vi "main.vi"() -> ()   [LabVIEW 2020]
uses:
  DataCluster.ctl
  <vilib>/userDefined/High Color/IMAQdx.ctl
  <vilib>/vision/Image Controls.llb/IMAQ Image.ctl
  <vilib>/Platform/TimedLoop/XDataNode/timing_clust.ctl
  <vilib>/Platform/TimedLoop/XDataNode/nitl_modes.ctl
  <vilib>/Platform/TimedLoop/XDataNode/wakeup.ctl
  <vilib>/DAQmx/write.llb/DAQmx Write (Analog DBL 1Chan 1Samp).vi
  <extravilib>/ChannelInstances/Tag-t'DataCluster.ctl'/Read With Abort.vi
  <extravilib>/ChannelInstances/Tag-c(a[.](dbl),a[.](dbl))/Write With Abort.vi
  <extravilib>/ChannelInstances/Tag-str/Write With Abort.vi
  <extravilib>/ChannelInstances/Tag-str/Read With Abort.vi
  <extravilib>/ChannelInstances/Tag-t'DataCluster.ctl'/Write With Abort.vi
  <extravilib>/ChannelInstances/Tag-c(a[.](dbl),a[.](dbl))/Instantiate.vi
  <extravilib>/ChannelInstances/Tag-str/Instantiate.vi
  <extravilib>/ChannelInstances/Tag-t'DataCluster.ctl'/Instantiate.vi
  <extravilib>/ChannelInstances/Tag-t'DataCluster.ctl'/EndpointRead.vi
  <extravilib>/ChannelInstances/Tag-c(a[.](dbl),a[.](dbl))/Endpoint.vi
  <extravilib>/ChannelInstances/Tag-str/Endpoint.vi
  <vilib>/DAQmx/create/channels.llb/DAQmx Create Channel (AI-Voltage-Basic).vi
  <vilib>/DAQmx/create/channels.llb/DAQmx Create Channel (AO-Voltage-Basic).vi
  <vilib>/DAQmx/miscellaneous.llb/DAQmx Fill In Error Info.vi
  <extravilib>/ChannelInstances/Tag-str/EndpointRead.vi
  <extravilib>/ChannelInstances/Tag-t'DataCluster.ctl'/Endpoint.vi
  <vilib>/platform/TimedLoop/XDataNode/XDataNode.xnode
  <vilib>/vision/driver/NI_Vision_Acquisition_Software.lvlib
  <extravilib>/ChannelInstances/Tag-t'DataCluster.ctl'.lvlib
  <vilib>/Platform/TimedLoop/XDataNode/XDNodeRunTimeDep.lvlib
  <resource>/objmgr/daqmx.rc
  <extravilib>/ChannelInstances/Tag-str.lvlib
  <extravilib>/ChannelInstances/Tag-c(a[.](dbl),a[.](dbl)).lvlib
panel:
  out "version":string="version 0.0.0.1" caption="Version"
  in  "Start":bool
  out "Title":string="Ice Nucleation Setup" caption="Version"
  in  "Help":bool
  out "Temps":waveform(dbl)[](graph)
  out "Gradients":waveform(dbl)[](graph)
  out "Camera Feed":T1(plugin-control)
  out "Period (ms)":i64
  out "Output%":dbl(slide) caption="Peltier Output" scale=0.0..100.0
  out "StatusString":string="Closing System"
  # "Camera Feed"
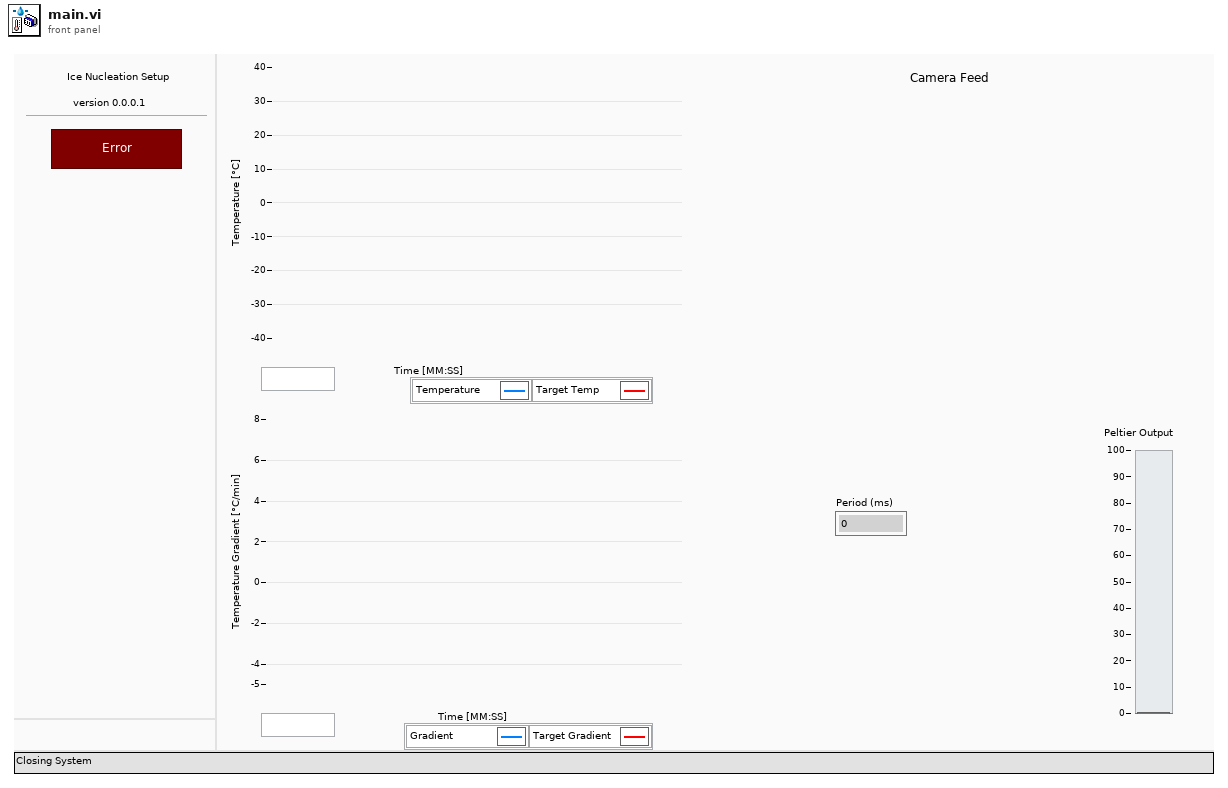
[diagram p1: front panel]
types:
  T1 = typedef "IMAQ Image.ctl" = refnum<image>
  T2 = typedef "DataCluster.ctl" = cluster{"Core":cluster{"Current VI Reference":refnum<vi>, "Close Panel on Exit?":bool, "Exit":bool}, "Connections":cluster{"cDAQ Therm":cluster{"Task":refnum<k21>, "Connected":bool, "Active":bool}, "cDAQ Voltage":cluster{"Task":refnum<k21>, "Connected":bool, "Active":bool}, "Camera":cluster{"Session":T3, "Connected":bool, "Active":bool}}, "Data Acquisition":cluster{"Setup":cluster{"Label":string, "Operator":string, "Notes":string, "TempGrad":dbl, "TargetTemp":dbl, "Sample Volume":dbl}, "Camera":cluster{"Image":T1, "Save Image":T1, "Image Frequency":i32, "Rectangle":T4}, "Thermistor":cluster{"Sample Size":i32, "Calibration":cluster{"B0.100":dbl[], "R25":dbl[], "c":dbl[][], "State":bool[], "V_S":dbl, "R_S":dbl}, "Timing Mode":i32}, "Partition":cluster{"Data":string[][], "Cell Label":string, "Cell Color":u32, "Height":i32, "Width":i32, "Grid":string[][]}, "Queue":cluster{"Size":i32, "Queue":refnum<queue>}, "Sample Rate":i32, "Active":bool, "Ready":bool, "Graph Mode":u16}, "Control":cluster{"Sample Rate":i32, "PID gains":cluster{"proportional gain (Kc)":dbl, "integral time (Ti, min)":dbl, "derivative time (Td, min)":dbl}}}
  T3 = typedef "IMAQdx.ctl" = refnum<k21>
  T4 = typedef "IMAQ Rectangle" = cluster{"Left":i32, "Top":i32, "Right":i32, "Bottom":i32, "Rotation":dbl}
  T5 = enum32{"Invalid", "Standard", "Closed", "Hidden", "Minimized", "Maximized"}
  T6 = enum32{"invalid app kind", "Development System", "Run Time System", "Student Edition", "Embedded LabVIEW", "Evaluation", "Custom"}
  T7 = cluster{"cDAQ Therm":cluster{"Task":refnum<k21>, "Connected":bool, "Active":bool}, "cDAQ Voltage":cluster{"Task":refnum<k21>, "Connected":bool, "Active":bool}, "Camera":cluster{"Session":T3, "Connected":bool, "Active":bool}}
  T8 = enum8{"Enabled", "Disabled", "Disabled and Grayed Out"}
  T9 = cluster{"Current VI Reference":refnum<vi>, "Close Panel on Exit?":bool, "Exit":bool}
  T10 = typedef "Tag-t'DataCluster.ctl'.lvlib/))Channel.ctl" = refnum<queue>
  T11 = typedef "XDNodeRunTimeDep.lvlib/timing_clust.ctl" = cluster{"Expected End [f-1]":u64, "Actual End [f-1]":u64, "Finished Late? [f-1]":bool, "Expected End [i-1]":u64, "Actual End [i-1]":u64, "Finished Late? [i-1]":bool, "Expected Start [i]":u64, "Actual Start [i]":u64, "Expected Start [f]":u64, "Actual Start [f]":u64, "Source Name":string, "Structure Name":string, "Period":i64, "Deadline":i64, "Offset":i64, "Start":i64, "Priority":i32, "Timeout":i32, "Mode":T12, "Wakeup Reason":T13, "Error":errorcluster, "Source Type":string, "Secondary Source Type":string, "Global End Time":u64, "Global Start Time":u64, "Frame Duration":u64, "Iteration Duration":u64, "Assigned CPU":i32, "I/O Scan Engine Mode":u32}
  T12 = typedef "XDNodeRunTimeDep.lvlib/nitl_modes.ctl" = enum32{"No Change", "Process missed periods, maintain original phase", "Discard missed periods, maintain original phase", "Process missed periods, ignore original phase", "Discard missed periods, ignore original phase"}
  T13 = typedef "XDNodeRunTimeDep.lvlib/wakeup.ctl" = enum32{"Normal", "Aborted", "Asynchronous wakeup", "Timing source error", "Timed loop error", "Timeout"}
  T14 = typedef "Tag-str.lvlib/))Channel.ctl" = refnum<queue>
  T15 = cluster{"Temperature Readings Duplicate":dbl[], "Voltage Readings Duplicate":dbl[]}
  T16 = typedef "Tag-c(a[.](dbl),a[.](dbl)).lvlib/))Channel.ctl" = refnum<queue>
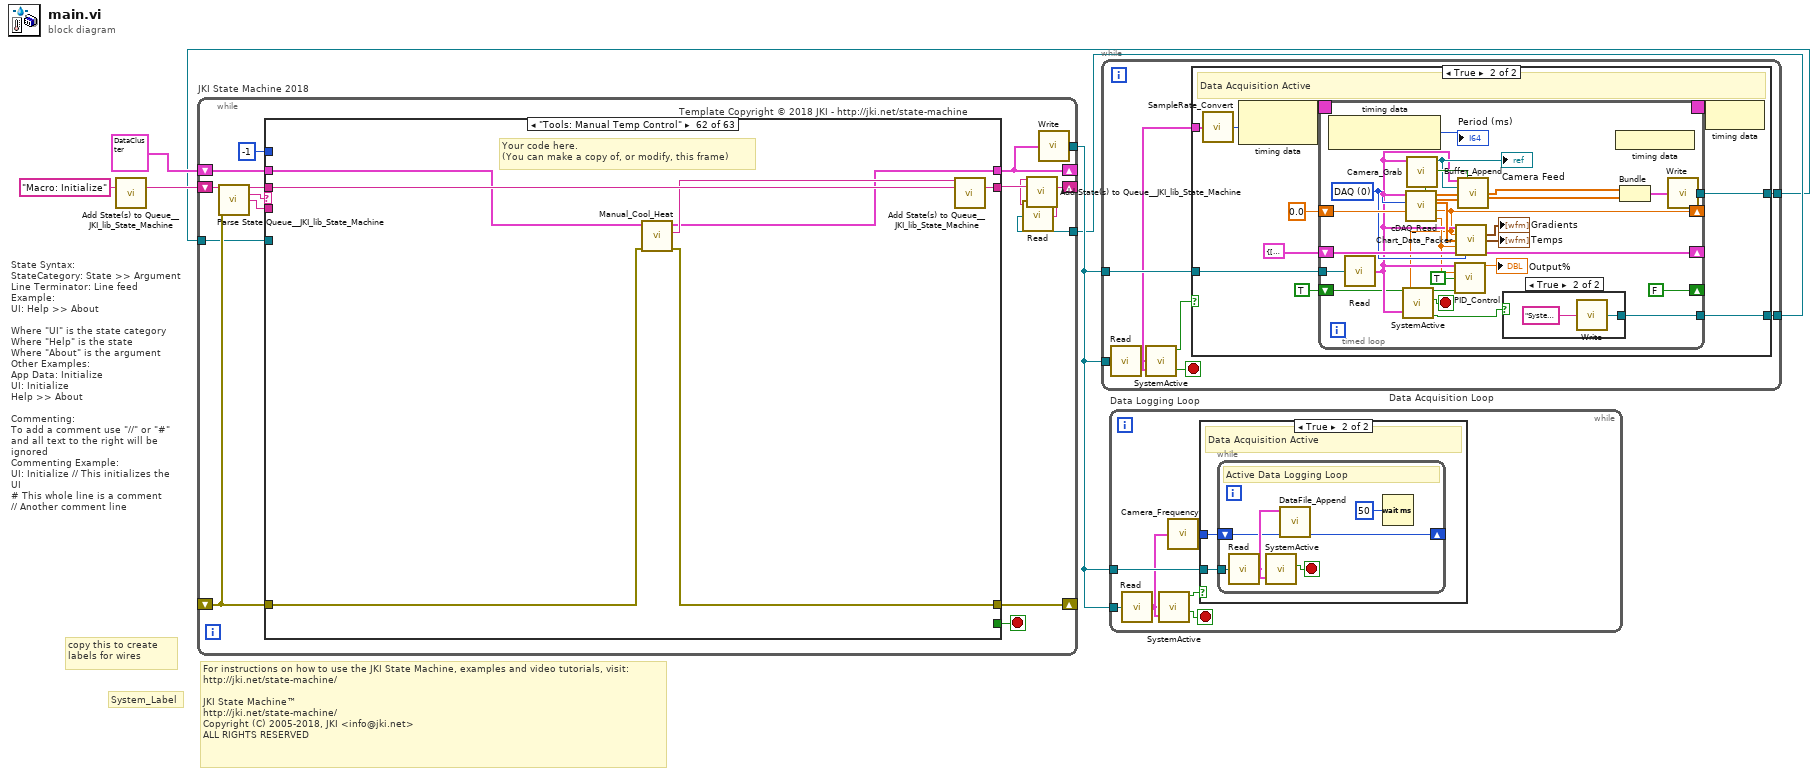
[diagram p0: block diagram]
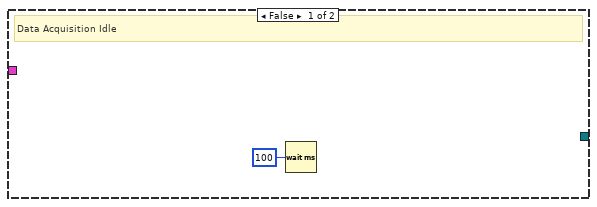
[diagram p2: hidden frame]
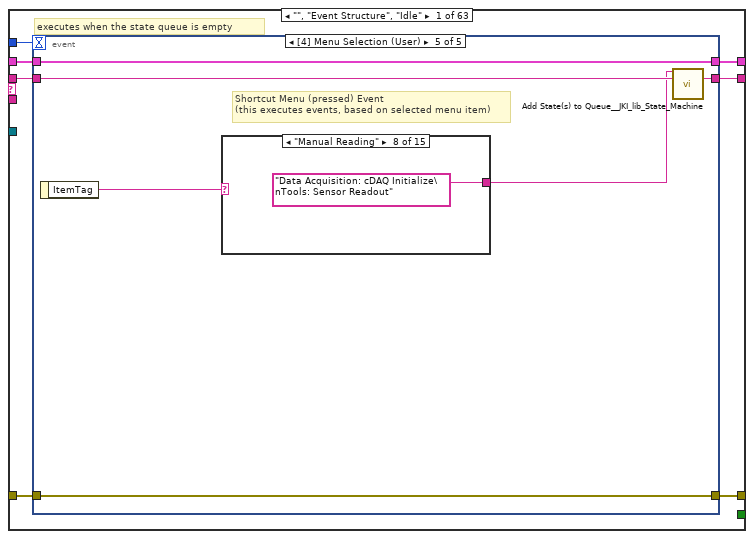
[diagram p4: hidden frame]
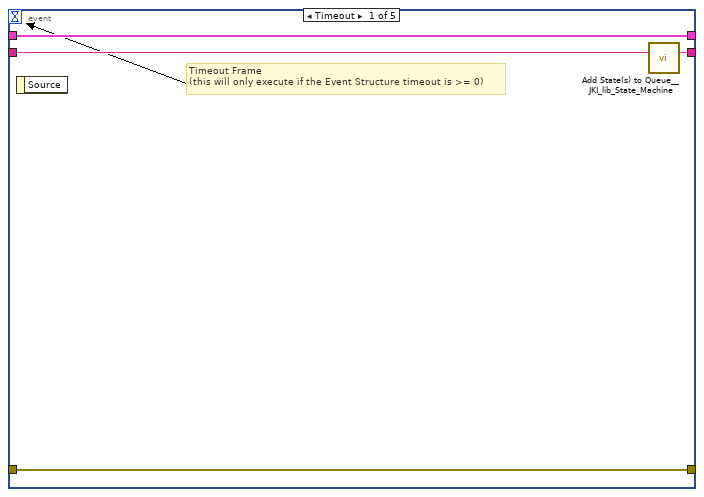
[diagram p5: hidden frame]
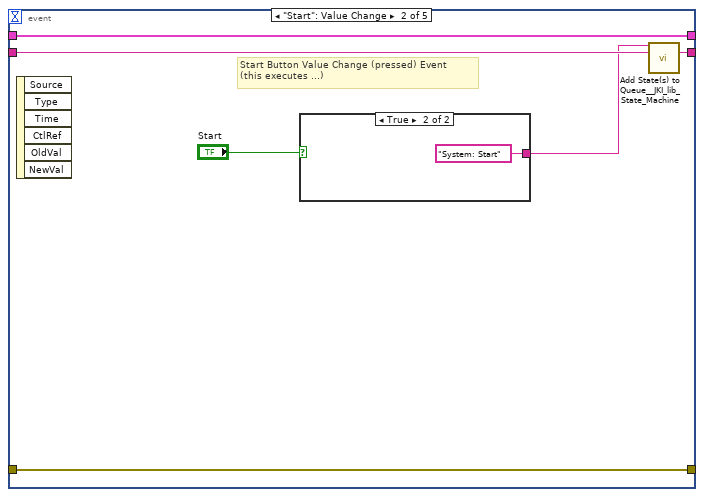
[diagram p6: hidden frame]
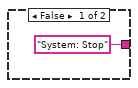
[diagram p7: hidden frame]
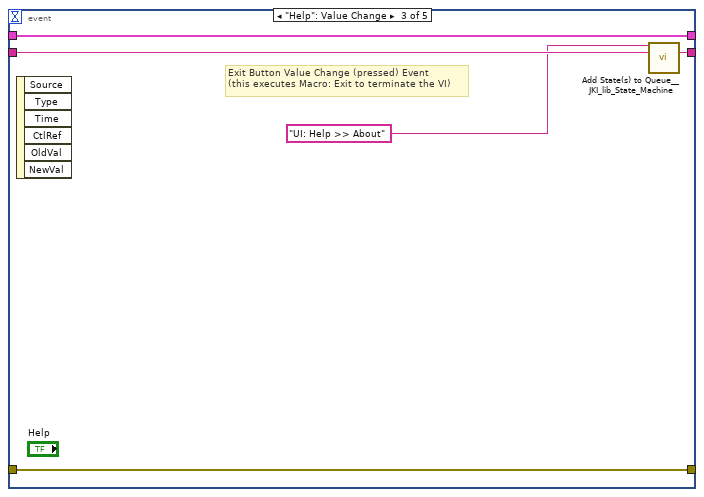
[diagram p8: hidden frame]
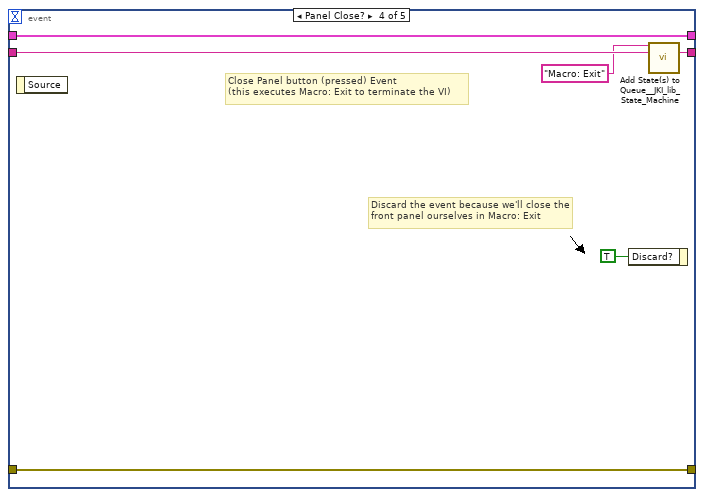
[diagram p9: hidden frame]
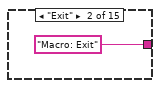
[diagram p11: hidden frame]
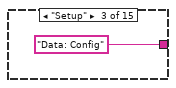
[diagram p12: hidden frame]
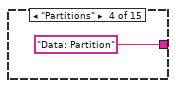
[diagram p13: hidden frame]
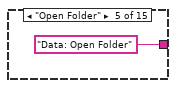
[diagram p14: hidden frame]
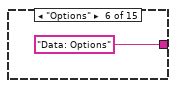
[diagram p15: hidden frame]
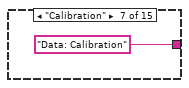
[diagram p16: hidden frame]
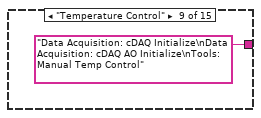
[diagram p17: hidden frame]
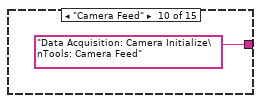
[diagram p18: hidden frame]
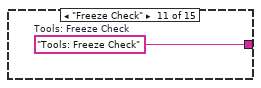
[diagram p19: hidden frame]
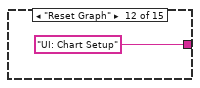
[diagram p20: hidden frame]
diagram:
  # "For instructions on how to use the JKI State Machine, examples and video tutorials, visit:\nhttp://jki.net/state-machine/\n\nJKI State Machine™\nhttp://jki.net/state-machine/\nCopyright (C) 2005-2018, JKI <info@jki.net>\nALL RIGHTS RESERVED"
  # "State Syntax:\nStateCategory: State >> Argument\nLine Terminator: Line feed\nExample:\nUI: Help >> About\n\nWhere \"UI\" is the state category\nWhere \"Help\" is the state\nWhere \"About\" is the argument\nOther Examples:\nApp Data: Initialize\nUI: Initialize\nHelp >> About\n\nCommenting:\nTo add a comment use \"//\" or \"#\" and all text to the right will be ignored\nCommenting Example:\nUI: Initialize // This initializes the UI\n# This whole line is a comment\n// Another comment line"
  # "copy this to create labels for wires"
  # "System_Label"
  n1 = call <vilib>:"Add State(s) to Queue__JKI_lib_State_Machine.vi"("State(s) in (\"\")"="Macro: Initialize") -> ("States Out"=w6:string)  [unwired: 14 in]
  n2 = while "JKI State Machine 2018" {
    shift-right: [w13] -> _
    shift-left: T2 {"Core"={"Current VI Reference"=refnum, "Close Panel on Exit?"=FALSE, "Exit"=FALSE}, "Connections"={"cDAQ Therm"={"Task"="", "Connected"=FALSE, "Active"=FALSE}, "cDAQ Voltage"={"Task"="", "Connected"=FALSE, "Active"=FALSE}, "Camera"={"Session"="", "Connected"=FALSE, "Active"=FALSE}}, "Data Acquisition"={"Setup"={"Label"="", "Operator"="", "Notes"="", "TempGrad"=0.0, "TargetTemp"=0.0, "Sample Volume"=1.0}, "Camera"={"Image"=refnum, "Save Image"=refnum, "Image Frequency"=20, "Rectangle"={"Left"=0, "Top"=0, "Right"=0, "Bottom"=0, "Rotation"=0.0}}, "Thermistor"={"Sample Size"=0, "Calibration"={"B0.100"=[], "R25"=[], "c"=[], "State"=[], "V_S"=0.0, "R_S"=0.0}, "Timing Mode"=14713}, "Partition"={"Data"=[], "Cell Label"="", "Cell Color"=0, "Height"=10, "Width"=16, "Grid"=[]}, "Queue"={"Size"=0, "Queue"=refnum}, "Sample Rate"=0, "Active"=FALSE, "Ready"=FALSE, "Graph Mode"=0}, "Control"={"Sample Rate"=0, "PID gains"={"proportional gain (Kc)"=0.0, "integral time (Ti, min)"=0.0, "derivative time (Td, min)"=0.0}}} ("DataCluster") -> [w16]
    shift-right: [w18] -> _
    shift-left: _ -> [w14]
    shift-right: [w10] -> _
    shift-left: w6 -> [w19]
    tunnel: [w12] -> w3
    tunnel: w2 -> [w9]
    tunnel: w1 -> [w7]
    stop <- w17 stop-if-true
    # "Template Copyright © 2018 JKI - http://jki.net/state-machine"
    n3 = call <vilib>:"Parse State Queue__JKI_lib_State_Machine.vi"("State Queue"=w19, "Error In (no error)"=w14) -> ("Remaining States"=w21:string, "Current State"=w22:string, "Arguments"=w20:string)  [unwired: 11 in]
    n4 = case shown="\"Tools: Manual Temp Control\"" w22 {
      selector: w22 -> [_ _ w77 _ _ _ _ _ _ _ _ _ _ _ _ _ _ _ _ _ _ _ _ _ _ _ _ _ _ _ _ _ _ _ _ _ _ _ _ _ _ _ _ _ _ _ _ _ _ _ _ _ _ _ _ _ _ _ _ _ _ _ _]
      tunnel: w21 -> [w29 w76 w81 w100 w106 w113 w117 w127 w134 w139 w144 w150 w156 w163 w168 w174 w180 w185 w209 w223 w238 w246 w251 w264 w282 w300 w314 w322 w338 w354 w372 w384 w394 w408 w413 w418 w423 w434 w442 w457 w468 w537 w542 w553 w557 w566 w579 w586 w596 w607 w623 w639 w655 w673 w689 w707 w714 w724 w737 w744 w750 w757 w761]
      tunnel: w20 -> [_ _ _ _ _ _ _ _ _ _ _ _ _ _ _ _ _ _ _ _ _ _ _ _ _ _ _ _ _ _ _ _ _ _ _ w414 w419 _ w438 w452 w462 _ _ _ _ _ _ _ _ _ _ _ _ _ _ _ _ _ _ _ _ _ _]
      tunnel: w16 -> [w27 w73 w79 w93 w103 w109 w114 _ w131 w136 w141 w148 w153 w161 w164 w172 w176 w183 w195 w217 w227 w243 w248 w254 w280 w298 w311 w318 w334 w350 w365 w381 w392 w406 w411 w416 w421 w431 w440 w455 w464 w534 w539 w550 w554 w558 w576 w581 w593 w602 w618 w634 w650 w668 w685 w705 w708 w715 w734 w742 w748 w755 w758]
      tunnel: [w26 w74 w83 w97 errorcluster {"status"=FALSE, "code"=0, "source"=""} ("error out") w111 w115 w118 w128 w137 w142 w145 w154 w158 w165 w170 w178 w181 w193 w210 w225 w244 w249 w261 w277 w296 w312 w315 w331 w347 w370 w382 w391 w405 w410 w415 w420 w432 w439 w453 w465 w535 w540 w551 w555 w564 w577 w584 w594 w603 w619 w635 w651 w669 w681 w703 w710 w717 w735 w740 w746 w753 w759] -> w18
      tunnel: w14 -> [w25 w74 w82 w97 w102 w111 w115 w119 w130 w137 w142 w145 w154 w159 w166 w171 w177 w182 w187 w211 w226 w244 w249 w260 w275 w295 w312 w316 w332 w348 w370 w382 w391 w405 w410 w415 w420 w432 w439 w454 w466 w535 w540 w551 w555 w564 w577 w584 w594 w604 w620 w636 w652 w670 w686 w704 w711 w717 w735 w741 w747 w754 w759]
      tunnel: [w28 w75 w80 w99 w105 w112 w116 w126 w133 w138 w143 w149 w155 w162 w167 w173 w179 w184 w208 w222 w237 w245 w250 w263 w281 w299 w313 w321 w337 w353 w371 w383 w393 w407 w412 w417 w422 w433 w441 w456 w467 w536 w541 w552 w556 w565 w578 w585 w595 w606 w622 w638 w654 w672 w688 w706 w713 w723 w736 w743 w749 w756 w760] -> w11
      tunnel: [_ _ _ _ _ TRUE _ _ _ _ _ _ _ _ _ _ _ _ _ _ _ _ _ _ _ _ _ _ _ _ _ _ _ _ _ _ _ _ _ _ _ _ _ _ _ _ _ _ _ _ _ _ _ _ _ _ _ _ _ _ _ _ _] -> w17
      tunnel: [w24 w73 w79 w98 w103 w107 w114 w125 w131 w135 w140 w147 w152 w160 w164 w169 w175 w183 w195 w217 w227 w243 w248 w262 w279 w297 w311 w317 w333 w349 w364 w381 w392 w406 w411 w416 w421 w431 w440 w455 w464 w534 w539 w550 w554 w558 w575 w580 w593 w601 w617 w633 w649 w671 w684 w702 w708 w719 w734 w742 w748 w751 w758] -> w13
      tunnel: -1 ("Timeout") -> [w23 _ _ _ _ _ _ _ _ _ _ _ _ _ _ _ _ _ _ _ _ _ _ _ _ _ _ _ _ _ _ _ _ _ _ _ _ _ _ _ _ _ _ _ _ _ _ _ _ _ _ _ _ _ _ _ _ _ _ _ _ _ _]
      tunnel: w7 -> [_ _ _ _ _ _ _ _ _ _ _ _ _ _ _ _ _ _ _ _ _ _ _ _ _ _ _ _ _ _ _ _ _ _ _ _ _ _ _ _ _ _ _ _ _ _ _ _ _ _ _ _ _ _ _ _ _ _ _ w739 _ _ _]
      frame "", "Event Structure", "Idle" {
        # "executes when the state queue is empty"
        n5 = event shown="[4] Menu Selection (User)" {
          selector: _ -> [_ _ _ _ _]
          dyn-events: _ -> [_ _ _ _ _]
          timeout: w23 -> [_ _ _ _ _]
          tunnel: w29 -> [w33 w39 w46 w52 w58]
          tunnel: [w32 w38 w45 w51 w57] -> w28
          tunnel: w27 -> [w30 w36 w43 w49 w55]
          tunnel: [w31 w37 w44 w50 w56] -> w26
          tunnel: w25 -> [w31 w37 w44 w50 w56]
          tunnel: [w30 w36 w43 w49 w55] -> w24
          event Timeout {
            # "Timeout Frame\n(this will only execute if the Event Structure timeout is >= 0)"
            n6 = event-data() -> ()  [unwired: 1 in, 1 out]
            n7 = call <vilib>:"Add State(s) to Queue__JKI_lib_State_Machine.vi"("State(s) in (\"\")"=w33) -> ("States Out"=w32:string)  [unwired: 14 in]
          }
          event "Start": Value Change {
            # "Start Button Value Change (pressed) Event\n(this executes ...)"
            n8 = event-data() -> ()  [unwired: 1 in, 6 out]
            n9 = case shown="True" "Start" {
              tunnel: ["System: Stop" ("State(s) in Front (\"\")") "System: Start" ("State(s) in Front (\"\")")] -> w34
              frame False {
              }
              frame True {
              }
            }
            n10 = call <vilib>:"Add State(s) to Queue__JKI_lib_State_Machine.vi"("State(s) in Front (\"\")"=w34, "State(s) in (\"\")"=w39) -> ("States Out"=w38:string)  [unwired: 13 in]
          }
          event "Help": Value Change {
            # "Exit Button Value Change (pressed) Event\n(this executes Macro: Exit to terminate the VI)"
            n11 = event-data() -> ()  [unwired: 1 in, 6 out]
            n12 = call <vilib>:"Add State(s) to Queue__JKI_lib_State_Machine.vi"("State(s) in Front (\"\")"="UI: Help >> About" ("State(s) in Front (\"\")"), "State(s) in (\"\")"=w46) -> ("States Out"=w45:string)  [unwired: 13 in]
          }
          event Panel Close? {
            # "Discard the event because we'll close the front panel ourselves in Macro: Exit"
            # "Close Panel button (pressed) Event\n(this executes Macro: Exit to terminate the VI)"
            n13 = event-data() -> ()  [unwired: 1 in, 1 out]
            n14 = event-data("Discard?"=TRUE) -> ()  [unwired: 1 in, 1 out]
            n15 = call <vilib>:"Add State(s) to Queue__JKI_lib_State_Machine.vi"("State(s) in Front (\"\")"="Macro: Exit", "State(s) in (\"\")"=w52) -> ("States Out"=w51:string)  [unwired: 13 in]
          }
          event Menu Selection (User) {
            # "Shortcut Menu (pressed) Event\n(this executes events, based on selected menu item)"
            n16 = event-data() -> ("ItemTag"=w54:string)  [unwired: 1 in]
            n17 = case shown="\"Manual Reading\"" w54 {
              tunnel: [_ "Macro: Exit" "Data: Config" "Data: Partition" "Data: Open Folder" "Data: Options" "Data: Calibration" "Data Acquisition: cDAQ Initialize\nTools: Sensor Readout" "Data Acquisition: cDAQ Initialize\nData Acquisition: cDAQ AO Initialize\nTools: Manual Temp Control" "Data Acquisition: Camera Initialize\nTools: Camera Feed" w68 "UI: Chart Setup" "UI: Cursor Set >> Busy\nConnections: Terminate\nConnections: Initialize\nUI: Cursor Set >> Idle" "System: Override" "UI: Connections Status"] -> w53
              frame "False", Default {
              }
              frame "Exit" {
              }
              frame "Setup" {
              }
              frame "Partitions" {
              }
              frame "Open Folder" {
              }
              frame "Options" {
              }
              frame "Calibration" {
              }
              frame "Manual Reading" {
              }
              frame "Temperature Control" {
              }
              frame "Camera Feed" {
              }
              frame "Freeze Check" {
                w68 = "Tools: Freeze Check"  # Tools: Freeze Check
              }
              frame "Reset Graph" {
              }
              frame "Reconnect" {
              }
              frame "System Override" {
              }
              frame "Status" {
              }
            }
            n18 = call <vilib>:"Add State(s) to Queue__JKI_lib_State_Machine.vi"("State(s) in Front (\"\")"=w53, "State(s) in (\"\")"=w58) -> ("States Out"=w57:string)  [unwired: 13 in]
          }
        }
      }
      frame "---------- Core ----------" {
        # "Do not put any code in this frame.\n(it is a separator no-op)"
        n19 = call <vilib>:"Add State(s) to Queue__JKI_lib_State_Machine.vi"("State(s) in (\"\")"=w76) -> ("States Out"=w75:string)  [unwired: 14 in]
      }
      frame Default {
        w86 = 42 items=["No error", "Argument error", "Memory is full", "Out of zone", "End of file", "File already open", "Generic file I/O error", "File not found", "File permission error", "Disk is full", "Duplicate path", "Too many files open", "System feature not enabled", "Resource file not found", "Cannot add resource", "Resource not found", "Image not found", "Image memory error", "Pen does not exist", "Config type invalid", "Config token not found", "Config parse error", "Config memory error", "Bad external code format", "Bad external code offset", "External code not present", "Null window", "Destroy window error", "Null menu", "Print aborted", "Bad print record", "Print driver error", "Windows error during printing", "Memory error during printing", "Print dialog error", "Generic print error", "Invalid device refnum", "Device not found", "Device parameter error", "Device unit error", "Cannot open device", "Device call aborted", "Generic error", "Cancelled by user", "Object ID too low", "Object ID too high", "Object not in heap", "Unknown heap", "Unknown object (invalid DefProc)", "Unknown object (DefProc not in table)", "Message out of range", "Invalid (null) method", "Unknown message", "Manager call not supported", "Bad address", "Network operation in progress", "Network operation timed out", "Connection is busy", "Network attribute not supported", "Network error", "Address in use", "System out of memory", "Connection aborted", "Connection refused", "Not connected", "Already connected", "Connection closed", "Initialization error (interapplication manager)", "Bad occurrence", "Wait on unbound occurrence handler", "Occurrence queue overflow", "Datalog type conflict", "Unused", "Unrecognized type (interapplication manager)", "Memory corrupt", "Failed to make temporary DLL", "Old CIN version", "Drag socket not found", "Failed to load drop-object", "Failed to register OLE object", "Failed to release OLE object", "Format specifier type mismatch", "Unknown format specifier", "Too few format specifiers", "Too many format specifiers", "Scan failed", "Newer CIN version", "Error converting to variant", "Runtime menu error", "Password tampered", "Variant attribute not found", "Incompatible variant data type", "Event data is not available", "Event Store is not present", "Occurrence is not found", "Event Queue is not created", "Event info is not available", "Refnum passed is NULL", "Error retrieving Class GUID", "Error retrieving CoClass GUID", "Error retrieving TypeLib GUID.", "Bad built application magic bytes.", "Specific driver is different from the specific driver associated with the Logical Name.", "There is no session opened to the class driver.", "Max Error", "MAX - Error with config objects", "MAX - Error loading configuration", "MAX - Group not supported"]
        # "Current State"
        # "Do not delete, rename, or modify this frame.\n(this is used to capture unhandled states and typos)"
        # "Handle mistyped state name (developer tool)"
        n20 = Format Into String(format string="Software Exception: Unhandled State \"%s\"." ("message"), error in=w82, w77) -> (resulting string=w85:string, error out=w84:errorcluster)  [unwired: 1 in]
        n21 = call <vilib>:"Error Cluster From Error Code.vi"("show call chain? (False)"=TRUE, "error in (no error)"=w84, "error message (\"\")"=w85, "error code (0)"=w86) -> ("error out"=w83:errorcluster)  [unwired: 5 in]
        n22 = call <vilib>:"Add State(s) to Queue__JKI_lib_State_Machine.vi"("State(s) in (\"\")"=w81) -> ("States Out"=w80:string)  [unwired: 14 in]
      }
      frame "Initialize Core Data" {
        # "Do not delete, rename, or modify this frame.\n(this is used to determine panel behavior on exit)"
        # "originally closed?"
        # "exe?"
        # "If panel starts closed or is an EXE, then close it when we exit"
        n23 = property class="VI"() -> ("FP.State"=w90:T5)  [unwired: 2 in, 2 out]
        n24 = property class="App"() -> ("App.Kind"=w96:T6)  [unwired: 2 in, 2 out]
        n25 = control-ref of="Current VI Reference"() -> (w91:refnum<vi>)
        n26 = Equal?(x=w90, y=T5."Closed" ("Front Panel Window:State")) -> (x = y?=w88:bool)
        n27 = Equal?(x=w96, y=T6."Run Time System" ("Application:Kind")) -> (x = y?=w94:bool)
        n28 = Or(x=w88, y=w94) -> (x .or. y?=w92:bool)
        n29 = Bundle By Name(cluster=w93, "Core.Current VI Reference"=w91, "Core.Close Panel on Exit?"=w92) -> (w98:T2)
        n30 = call <vilib>:"Add State(s) to Queue__JKI_lib_State_Machine.vi"("State(s) in (\"\")"=w100) -> ("States Out"=w99:string)  [unwired: 14 in]
      }
      frame "Error Handler" {
        # "Unhandled Error -- Display it"
        # "Handle any errors here.\nYou can also output any states to clean-up after errors occur"
        # "Clear error"
        n31 = call <vilib>:"General Error Handler.vi"("error in (no error)"=w102) -> ()  [unwired: 10 in, 5 out]
        n32 = call <vilib>:"Add State(s) to Queue__JKI_lib_State_Machine.vi"("State(s) in Front (\"\")"="/* Post Error States", "State(s) in (\"\")"=w106) -> ("States Out"=w105:string)  [unwired: 13 in]
      }
      frame "Exit" {
        # "Do not put any code in this frame.\n(No errors that occur here will be handled.)"
        n33 = Bundle By Name(cluster=w109, "Core.Exit"=TRUE) -> (w107:T2)
        n34 = call <vilib>:"Add State(s) to Queue__JKI_lib_State_Machine.vi"("State(s) in (\"\")"=w113) -> ("States Out"=w112:string)  [unwired: 14 in]
      }
      frame "---------- Data ----------" {
        # "Do not put any code in this frame.\n(It is a separator no-op. You can make a copy of this frame to create a new Data frame)"
        n35 = call <vilib>:"Add State(s) to Queue__JKI_lib_State_Machine.vi"("State(s) in (\"\")"=w117) -> ("States Out"=w116:string)  [unwired: 14 in]
      }
      frame "Data: Initialize" {
        w124 = T9 {"Current VI Reference"=refnum, "Close Panel on Exit?"=FALSE, "Exit"=FALSE}  # Core
        # "Initialize the shift-register data, here.\n(data names are defined by what you wire into the bundle function)"
        n36 = call "Settings_Load.vi"("error in"=w119) -> ("error out"=w120:errorcluster, "DataCluster out"=w121:T2)  [unwired: 9 in]
        n37 = call "Settings_Save.vi"("error in"=w120, "DataCluster"=w121) -> ("error out"=w118:errorcluster)  [unwired: 9 in]
        n38 = Bundle By Name(cluster=w121, "Core"=w124, "Connections"=T7 {"cDAQ Therm"={"Task"="ThermTask", "Connected"=FALSE, "Active"=FALSE}, "cDAQ Voltage"={"Task"="", "Connected"=FALSE, "Active"=FALSE}, "Camera"={"Session"="", "Connected"=FALSE, "Active"=FALSE}}, "Data Acquisition.Active"=FALSE ("System.Active")) -> (w125:T2)
        n39 = call <vilib>:"Add State(s) to Queue__JKI_lib_State_Machine.vi"("State(s) in (\"\")"=w127) -> ("States Out"=w126:string)  [unwired: 14 in]
      }
      frame "Data: Cleanup" {
        # "Cleanup any data and references, here.\n(this is called automatically, by the Macro: Exit)"
        n40 = Unbundle By Name(w131) -> ("Core.Current VI Reference"=w132:refnum<vi>)
        n41 = call "Settings_Save.vi"("error in"=w130, "DataCluster"=w131) -> ("error out"=w129:errorcluster)  [unwired: 9 in]
        n42 = Close Reference(reference=w132, error in (no error)=w129) -> (error out=w128:errorcluster)
        n43 = call <vilib>:"Add State(s) to Queue__JKI_lib_State_Machine.vi"("State(s) in (\"\")"=w134) -> ("States Out"=w133:string)  [unwired: 14 in]
      }
      frame "Data: Config" {
        # "Access Data Setup here.\n(this is called automatically, by the Settings Event Run time menu)"
        n44 = call "Settings_Config.vi"("DataCluster in"=w136) -> ("DataCluster out"=w135:T2)  [unwired: 10 in]
        n45 = call <vilib>:"Add State(s) to Queue__JKI_lib_State_Machine.vi"("State(s) in (\"\")"=w139) -> ("States Out"=w138:string)  [unwired: 14 in]
      }
      frame "Data: Partition" {
        # "Access Data Setup here.\n(this is called automatically, by the Settings Event Run time menu)"
        n46 = call "Partition_Setup.vi"("DataCluster in"=w141) -> ("DataCluster out"=w140:T2)  [unwired: 9 in, 1 out]
        n47 = call <vilib>:"Add State(s) to Queue__JKI_lib_State_Machine.vi"("State(s) in (\"\")"=w144) -> ("States Out"=w143:string)  [unwired: 14 in]
      }
      frame "Data: Options" {
        # "Access Data Setup here.\n(this is called automatically, by the Settings Event Run time menu)"
        n48 = call "Options.vi"("DataCluster in"=w148) -> ("State"=w146:string, "DataCluster out"=w147:T2)  [unwired: 9 in]
        n49 = call <vilib>:"Add State(s) to Queue__JKI_lib_State_Machine.vi"("State(s) in Front (\"\")"=w146, "State(s) in (\"\")"=w150) -> ("States Out"=w149:string)  [unwired: 13 in]
      }
      frame "Data: Calibration" {
        # "Access Data Setup here.\n(this is called automatically, by the Settings Event Run time menu)"
        n50 = call "Thermistor_Callibration.vi"("DataCluster in"=w153) -> ("State Out"=w151:string, "DataCluster out"=w152:T2)  [unwired: 9 in]
        n51 = call <vilib>:"Add State(s) to Queue__JKI_lib_State_Machine.vi"("State(s) in Front (\"\")"=w151, "State(s) in (\"\")"=w156) -> ("States Out"=w155:string)  [unwired: 13 in]
      }
      frame "Data: Load Calibration" {
        # "Access Data Setup here.\n(this is called automatically, by the Settings Event Run time menu)"
        n52 = call "Thermistor_Callibration_Load.vi"("error in"=w159, "DataCluster"=w161) -> ("error out"=w158:errorcluster, "State"=w157:string, "DataCluster out"=w160:T2)  [unwired: 7 in]
        n53 = call <vilib>:"Add State(s) to Queue__JKI_lib_State_Machine.vi"("State(s) in Front (\"\")"=w157, "State(s) in (\"\")"=w163) -> ("States Out"=w162:string)  [unwired: 13 in]
      }
      frame "Data: Save Calibration" {
        # "Access Data Setup here.\n(this is called automatically, by the Settings Event Run time menu)"
        n54 = call "Thermistor_Callibration_Save.vi"("error in"=w166, "DataCluster"=w164) -> ("error out"=w165:errorcluster)  [unwired: 9 in]
        n55 = call <vilib>:"Add State(s) to Queue__JKI_lib_State_Machine.vi"("State(s) in (\"\")"=w168) -> ("States Out"=w167:string)  [unwired: 14 in]
      }
      frame "Data: Setup File Config" {
        # "Access Data Setup here.\n(this is called automatically, by the Settings Event Run time menu)"
        n56 = call "SetupFile_Create.vi"("error in (no error)"=w171, "DataCluster"=w172) -> ("error out"=w170:errorcluster, "DataCluster out"=w169:T2)  [unwired: 8 in]
        n57 = call <vilib>:"Add State(s) to Queue__JKI_lib_State_Machine.vi"("State(s) in (\"\")"=w174) -> ("States Out"=w173:string)  [unwired: 14 in]
      }
      frame "Data: Stamp times" {
        # "Access Data Setup here.\n(this is called automatically, by the Settings Event Run time menu)"
        n58 = call "SetupFile_Stamp.vi"("error in (no error)"=w177, "DataCluster"=w176) -> ("error out"=w178:errorcluster, "DataCluster out"=w175:T2)  [unwired: 8 in]
        n59 = call <vilib>:"Add State(s) to Queue__JKI_lib_State_Machine.vi"("State(s) in (\"\")"=w180) -> ("States Out"=w179:string)  [unwired: 14 in]
      }
      frame "Data: Data File Config" {
        # "Access Data Setup here.\n(this is called automatically, by the Settings Event Run time menu)"
        n60 = call "DataFile_Create.vi"("error in (no error)"=w182, "DataCluster"=w183) -> ("error out"=w181:errorcluster)  [unwired: 9 in]
        n61 = call <vilib>:"Add State(s) to Queue__JKI_lib_State_Machine.vi"("State(s) in (\"\")"=w185) -> ("States Out"=w184:string)  [unwired: 14 in]
      }
      frame "Data: Files Unlock" {
        # "Access Data Setup here.\n(this is called automatically, by the Settings Event Run time menu)"
        n62 = Unbundle By Name(w195) -> ("Data Acquisition.Setup.Label"=w203:string)
        n63 = call <vilib>:"Application Directory.vi"() -> ("Application Directory"=w201:path)
        n64 = Path To String(path=w201) -> (string=w202:string)
        n65 = Concatenate Strings(w202, "\\Data\\", w203) -> (w188:string)
        n66 = Concatenate Strings(w188, "\\Partition.csv") -> (w191:string)
        n67 = Concatenate Strings(w188, "\\Setup.csv") -> (w205:string)
        n68 = Concatenate Strings(w188, "\\Data.csv") -> (w204:string)
        n69 = String To Path(string=w191) -> (path=w192:path)
        n70 = String To Path(string=w205) -> (path=w206:path)
        n71 = String To Path(string=w204) -> (path=w207:path)
        n72 = Set Permissions(7:i16 448 ("permissions"), 8:w187, 11:w192) -> (0:w186:errorcluster)  [unwired: 2 in, 1 out]
        n73 = Set Permissions(7:i16 448 ("permissions"), 8:w186, 11:w207) -> (0:w194:errorcluster)  [unwired: 2 in, 1 out]
        n74 = Set Permissions(7:i16 448 ("permissions"), 8:w194, 11:w206) -> (0:w193:errorcluster)  [unwired: 2 in, 1 out]
        n75 = call <vilib>:"Add State(s) to Queue__JKI_lib_State_Machine.vi"("State(s) in (\"\")"=w209) -> ("States Out"=w208:string)  [unwired: 14 in]
      }
      frame "Data: Open Folder" {
        # "Access Data Setup here.\n(this is called automatically, by the Settings Event Run time menu)"
        n76 = Unbundle By Name(w217) -> ("Data Acquisition.Setup.Label"=w221:string)
        n77 = call <vilib>:"Application Directory.vi"() -> ("Application Directory"=w219:path)
        n78 = Path To String(path=w219) -> (string=w220:string)
        n79 = Concatenate Strings(w220, "\\Data\\", w221) -> (w216:string)
        n80 = String To Path(string=w216) -> (path=w214:path)
        n81 = Format Into String(format string="cmd /c explorer.exe \"%s\"", w214) -> (resulting string=w213:string)  [unwired: 2 in, 1 out]
        n82 = call <vilib>:"System Exec.vi"("run minimized? (F)"=TRUE, "error in (no error)"=w211, "command line"=w213) -> ("error out"=w210:errorcluster)  [unwired: 5 in, 3 out]
        n83 = call <vilib>:"Add State(s) to Queue__JKI_lib_State_Machine.vi"("State(s) in (\"\")"=w223) -> ("States Out"=w222:string)  [unwired: 14 in]
      }
      frame "Data: Image Folder Setup" {
        # "Access Data Setup here.\n(this is called automatically, by the Settings Event Run time menu)"
        n84 = Unbundle By Name(w227) -> ("Data Acquisition.Setup.Label"=w229:string)
        n85 = call <vilib>:"Application Directory.vi"() -> ("Application Directory"=w236:path)
        n86 = Path To String(path=w236) -> (string=w235:string)
        n87 = Concatenate Strings(w235, "\\Data\\", w229, "\\Images\\" ("string")) -> (w233:string)
        n88 = String To Path(string=w233) -> (path=w232:path)
        n89 = call <vilib>:"Check if File or Folder Exists.vi"("error in (no error)"=w226, "path"=w232) -> ("error out"=w228:errorcluster, "file or folder exists?"=w231:bool, "dup path"=w230:path)  [unwired: 7 in]
        n90 = case shown="False" w231 {
          tunnel: w230 -> [w241 _]
          tunnel: w228 -> [w240 w242]
          tunnel: [w239 w242] -> w225
          frame False {
            n91 = Create Folder(path (use dialog)=w241, error in=w240) -> (error out=w239:errorcluster)  [unwired: 1 in, 2 out]
          }
          frame True {
          }
        }
        n92 = call <vilib>:"Add State(s) to Queue__JKI_lib_State_Machine.vi"("State(s) in (\"\")"=w238) -> ("States Out"=w237:string)  [unwired: 14 in]
      }
      frame "---------- Connections ----------" {
        # "Do not put any code in this frame.\n(It is a separator no-op. You can make a copy of this frame to create a new Data frame)"
        n93 = call <vilib>:"Add State(s) to Queue__JKI_lib_State_Machine.vi"("State(s) in (\"\")"=w246) -> ("States Out"=w245:string)  [unwired: 14 in]
      }
      frame "Connections: Initialize" {
        # "Initialize the System Connections, here.\n(this is called automatically, by the Macro: Init)"
        n94 = call <vilib>:"Add State(s) to Queue__JKI_lib_State_Machine.vi"("State(s) in Front (\"\")"="UI: StatusString >> Connecting cDAQ (Thermistors)\nConnections: Initialize cDAQ Therm\nUI: StatusString >> Connecting cDAQ Connection (Voltage Control)\nConnections: Initialize cDAQ AO\nUI: StatusString >> Connecting Camera\nConnections: Initialize Camera\nUI: StatusString >> Validating Connections\nConnections: Status" ("State(s) in Front (\"\")"), "State(s) in (\"\")"=w251) -> ("States Out"=w250:string)  [unwired: 13 in]
      }
      frame "Connections: Initialize cDAQ Therm" {
        w259 = 10106 items=["Default"=-1, "RSE"=10083, "NRSE"=10078, "Differential"=10106, "Pseudodifferential"=12529] ("input terminal configuration")
        # "Setup connection to cDAQs"
        # "Initialize the System Connections, here.\n(this is called automatically, by the Macro: Init)"
        n95 = Unbundle By Name(w254) -> ("Data Acquisition.Thermistor.Timing Mode"=w253:i32)
        n96 = call-poly <vilib>:"DAQmx Create Virtual Channel.vi"("input terminal configuration"=w259, "physical channels"="cDAQ1Mod2/ai3:0, cDAQ1Mod3/ai3:0", "error in"=w260) -> ("task out"=w258:refnum<k21>, "error out"=w257:errorcluster)  [unwired: 11 in]
        n97 = property class="DAQmx Channel"(reference=w258, error in=w257, "AI.ADCTimingMode"=w253) -> (reference out=w255:refnum<k21>, error out=w256:errorcluster)
        n98 = case shown="No Error" w256 {
          selector: w256 -> [w265 _]
          tunnel: w254 -> [w269 w273]
          tunnel: [w268 w272] -> w262
          tunnel: w255 -> [w266 _]
          tunnel: [w265 errorcluster {"status"=FALSE, "code"=0, "source"=""} ("error IO")] -> w261
          frame No Error {
            n99 = Bundle By Name(cluster=w269, "Connections.cDAQ Therm.Task"=w266, "Connections.cDAQ Therm.Connected"=TRUE ("Connections.cDAQ.Connected")) -> (w268:T2)
          }
          frame Error {
            n100 = Bundle By Name(cluster=w273, "Connections.cDAQ Therm.Connected"=FALSE ("Connections.cDAQ.Connected")) -> (w272:T2)
          }
        }
        n101 = call <vilib>:"Add State(s) to Queue__JKI_lib_State_Machine.vi"("State(s) in (\"\")"=w264) -> ("States Out"=w263:string)  [unwired: 14 in]
      }
      frame "Connections: Initialize cDAQ AO" {
        # "Setup connection to cDAQs"
        # "Initialize the System Connections, here.\n(this is called automatically, by the Macro: Init)"
        n102 = call-poly <vilib>:"DAQmx Create Virtual Channel.vi"("physical channels"="cDAQ1Mod1/ao0", "error in"=w275) -> ("task out"=w278:refnum<k21>, "error out"=w274:errorcluster)  [unwired: 12 in]
        n103 = case shown="Error .." w274 {
          selector: w274 -> [w283 _]
          tunnel: w280 -> [w287 w291]
          tunnel: [w286 w290] -> w279
          tunnel: w278 -> [w284 _]
          tunnel: [w283 errorcluster {"status"=FALSE, "code"=0, "source"=""} ("error IO")] -> w277
          frame No Error {
            n104 = Bundle By Name(cluster=w287, "Connections.cDAQ Voltage.Task"=w284, "Connections.cDAQ Voltage.Connected"=TRUE ("Connections.cDAQ.Connected")) -> (w286:T2)
          }
          frame Error {
            n105 = Bundle By Name(cluster=w291, "Connections.cDAQ Voltage.Connected"=FALSE ("Connections.cDAQ.Connected")) -> (w290:T2)
          }
        }
        n106 = call <vilib>:"Add State(s) to Queue__JKI_lib_State_Machine.vi"("State(s) in (\"\")"=w282) -> ("States Out"=w281:string)  [unwired: 14 in]
      }
      frame "Connections: Initialize Camera" {
        # "Setup connection to cDAQs"
        # "Initialize the System Connections, here.\n(this is called automatically, by the Macro: Init)"
        n107 = call <vilib>:"IMAQdx Open Camera.vi"("error in"=w295, "Session In"="16511205") -> ("error out"=w294:errorcluster, "Session Out"=w293:T3)  [unwired: 8 in]
        n108 = case shown="Error .." w294 {
          selector: w294 -> [w302 _]
          tunnel: w298 -> [w305 w309]
          tunnel: [w304 w308] -> w297
          tunnel: [w302 errorcluster {"status"=FALSE, "code"=0, "source"=""} ("error IO")] -> w296
          tunnel: w293 -> [w301 _]
          frame No Error {
            n109 = Bundle By Name(cluster=w305, "Connections.Camera.Session"=w301, "Connections.Camera.Connected"=TRUE ("Connections.cDAQ.Connected")) -> (w304:T2)
          }
          frame Error {
            n110 = Bundle By Name(cluster=w309, "Connections.Camera.Connected"=FALSE ("Connections.cDAQ.Connected")) -> (w308:T2)
          }
        }
        n111 = call <vilib>:"Add State(s) to Queue__JKI_lib_State_Machine.vi"("State(s) in (\"\")"=w300) -> ("States Out"=w299:string)  [unwired: 14 in]
      }
      frame "Connections: Terminate" {
        # "Terminate connection to DAQs and Power Supply (Peltier)"
        # "Terminate the System Connections, here.\n(this is called automatically, by the Macro: Exit)"
        n112 = call <vilib>:"Add State(s) to Queue__JKI_lib_State_Machine.vi"("State(s) in Front (\"\")"="UI: StatusString >> Terminating cDAQ Connection (Thermistors)\nConnections: Terminate cDAQ Therm\nUI: StatusString >> Terminating cDAQ Connection (Voltage Control)\nConnections: Terminate cDAQ AO\nUI: StatusString >> Terminating Camera Connection\nConnections: Terminate Camera" ("State(s) in Front (\"\")"), "State(s) in (\"\")"=w314) -> ("States Out"=w313:string)  [unwired: 13 in]
      }
      frame "Connections: Terminate cDAQ Therm" {
        # "Terminate connection to DAQs and Power Supply (Peltier)"
        # "Terminate the System Connections, here.\n(this is called automatically, by the Macro: Exit)"
        n113 = Unbundle By Name(w318) -> ("Connections.cDAQ Therm.Task"=w319:refnum<k21>, "Connections.cDAQ Therm.Connected"=w320:bool)
        n114 = case shown="True" w320 {
          tunnel: w319 -> [_ w330]
          tunnel: w318 -> [w324 w329]
          tunnel: [w324 w327] -> w317
          tunnel: w316 -> [w323 w326]
          tunnel: [w323 w325] -> w315
          frame False {
          }
          frame True {
            n115 = call <vilib>:"DAQmx Clear Task.vi"("task in"=w330, "error in"=w326) -> ("error out"=w325:errorcluster)  [unwired: 13 in]
            n116 = Bundle By Name(cluster=w329, "Connections.cDAQ Therm.Connected"=FALSE ("Connections.cDAQ.Connected")) -> (w327:T2)
          }
        }
        n117 = call <vilib>:"Add State(s) to Queue__JKI_lib_State_Machine.vi"("State(s) in (\"\")"=w322) -> ("States Out"=w321:string)  [unwired: 14 in]
      }
      frame "Connections: Terminate cDAQ AO" {
        # "Terminate connection to DAQs and Power Supply (Peltier)"
        # "Terminate the System Connections, here.\n(this is called automatically, by the Macro: Exit)"
        n118 = Unbundle By Name(w334) -> ("Connections.cDAQ Voltage.Task"=w335:refnum<k21>, "Connections.cDAQ Voltage.Connected"=w336:bool)
        n119 = case shown="True" w336 {
          tunnel: w335 -> [_ w346]
          tunnel: w334 -> [w340 w345]
          tunnel: [w340 w343] -> w333
          tunnel: w332 -> [w339 w342]
          tunnel: [w339 w341] -> w331
          frame False {
          }
          frame True {
            n120 = call <vilib>:"DAQmx Clear Task.vi"("task in"=w346, "error in"=w342) -> ("error out"=w341:errorcluster)  [unwired: 13 in]
            n121 = Bundle By Name(cluster=w345, "Connections.cDAQ Voltage.Connected"=FALSE ("Connections.cDAQ.Connected")) -> (w343:T2)
          }
        }
        n122 = call <vilib>:"Add State(s) to Queue__JKI_lib_State_Machine.vi"("State(s) in (\"\")"=w338) -> ("States Out"=w337:string)  [unwired: 14 in]
      }
      frame "Connections: Terminate Camera" {
        # "Terminate connection to DAQs and Power Supply (Peltier)"
        # "Terminate the System Connections, here.\n(this is called automatically, by the Macro: Exit)"
        n123 = Unbundle By Name(w350) -> ("Connections.Camera.Session"=w351:T3, "Connections.Camera.Connected"=w352:bool)
        n124 = case shown="False" w352 {
          tunnel: w351 -> [_ w359]
          tunnel: w350 -> [w356 w362]
          tunnel: [w356 w360] -> w349
          tunnel: w348 -> [w355 w358]
          tunnel: [w355 w357] -> w347
          frame False {
          }
          frame True {
            n125 = call <vilib>:"IMAQdx Close Camera.vi"("error in"=w358, "Session In"=w359) -> ("error out"=w357:errorcluster)  [unwired: 9 in]
            n126 = Bundle By Name(cluster=w362, "Connections.cDAQ Therm.Connected"=FALSE ("Connections.cDAQ.Connected")) -> (w360:T2)
          }
        }
        n127 = call <vilib>:"Add State(s) to Queue__JKI_lib_State_Machine.vi"("State(s) in (\"\")"=w354) -> ("States Out"=w353:string)  [unwired: 14 in]
      }
      frame "Connections: Status" {
        # "Checks Connection Status , here.\n(this is called automatically, by the Connections: Initialize)"
        n128 = Unbundle By Name(w365) -> ("Connections.cDAQ Therm.Connected"=w368:bool, "Connections.cDAQ Voltage.Connected"=w367:bool, "Connections.Camera.Connected"=w363:bool)
        n129 = Compound Arithmetic op=AND(w368, w367, w363) -> (w369:bool)
        n130 = case shown="True" w369 {
          selector: w369 -> [w373 w378]
          tunnel: ["UI: Start Button >> Error\nUI: StatusString >> Connection Error!" "UI: Start Button >> Default\nUI: StatusString >> Idle"] -> w366
          tunnel: w365 -> [w375 w379]
          tunnel: [w374 w377] -> w364
          frame False {
            n131 = Bundle By Name(cluster=w375, "Data Acquisition.Ready"=w373) -> (w374:T2)
          }
          frame True {
            n132 = Bundle By Name(cluster=w379, "Data Acquisition.Ready"=w378) -> (w377:T2)
          }
        }
        n133 = call <vilib>:"Add State(s) to Queue__JKI_lib_State_Machine.vi"("State(s) in Front (\"\")"=w366, "State(s) in (\"\")"=w372) -> ("States Out"=w371:string)  [unwired: 13 in]
      }
      frame "---------- UI ----------" {
        # "Do not put any code in this frame.\n(It is a separator no-op. You can make a copy of this frame to create a new UI frame)"
        n134 = call <vilib>:"Add State(s) to Queue__JKI_lib_State_Machine.vi"("State(s) in (\"\")"=w384) -> ("States Out"=w383:string)  [unwired: 14 in]
      }
      frame "UI: Initialize" {
        # "Initialize the User Interface, here.\n(this is called automatically, by the Macro: Init)"
        n135 = local write "Start"(FALSE ("Start")) -> ()
        n136 = call "Read Exe Version.vi"() -> ("FileVersion"=w388:string)  [unwired: 10 in, 1 out]
        n137 = Concatenate Strings("version " ("string"), w388) -> (→"version":string)
        n138 = call <vilib>:"Add State(s) to Queue__JKI_lib_State_Machine.vi"("State(s) in Front (\"\")"="UI: StatusString >> Clearing Chart History\nUI: Chart Setup\nUI: Chart Clear" ("State(s) in Front (\"\")"), "State(s) in (\"\")"=w394) -> ("States Out"=w393:string)  [unwired: 13 in]
        "Title" <- "Ice Nucleation Setup" ("Version")
      }
      frame "UI: Chart Setup" {
        # "Initialize the User Interface, here.\n(this is called automatically, by the Macro: Init)"
        n139 = property on="Temps" class="WFChart (strict)"("XScale.Maximum"=300.0 ("X Scale.Range:Maximum"), "XScale.Minimum"=0.0 ("X Scale.Range:Minimum"), "ActYScl"=0 ("Active Y Scale"), "YScale.Maximum"=40.0 ("X Scale.Range:Maximum"), "YScale.Minimum"=-40.0 ("X Scale.Range:Minimum")) -> ()  [unwired: 2 in, 2 out]
        n140 = property on="Temps" class="WFChart (strict)"("XScale.Maximum"=300.0 ("X Scale.Range:Maximum"), "XScale.Minimum"=0.0 ("X Scale.Range:Minimum"), "ActYScl"=0 ("Active Y Scale"), "YScale.Maximum"=8.0 ("Y Scale.Range:Maximum"), "YScale.Minimum"=-5.0 ("Y Scale.Range:Minimum")) -> ()  [unwired: 2 in, 2 out]
        n141 = call <vilib>:"Add State(s) to Queue__JKI_lib_State_Machine.vi"("State(s) in (\"\")"=w408) -> ("States Out"=w407:string)  [unwired: 14 in]
      }
      frame "UI: Chart Clear" {
        w409 = waveform(dbl)[][] [] ("History Data")
        # "Initialize the User Interface, here.\n(this is called automatically, by the Macro: Init)"
        n142 = property on="Temps" class="WFChart (strict)"("History Data"=w409) -> ()  [unwired: 2 in, 2 out]
        n143 = property on="Gradients" class="WFChart (strict)"("History Data"=w409) -> ()  [unwired: 2 in, 2 out]
        n144 = call <vilib>:"Add State(s) to Queue__JKI_lib_State_Machine.vi"("State(s) in (\"\")"=w413) -> ("States Out"=w412:string)  [unwired: 14 in]
      }
      frame "UI: StatusString" {
        # "Argument"
        # "Set Status String here\n(this is called takes argument and applies to Status String)"
        n145 = call <vilib>:"Add State(s) to Queue__JKI_lib_State_Machine.vi"("State(s) in (\"\")"=w418) -> ("States Out"=w417:string)  [unwired: 14 in]
        "StatusString" <- w414
      }
      frame "UI: Help" {
        # "Argument"
        # "Set Status String here\n(this is called takes argument and applies to Status String)"
        n146 = case shown="\"About\"" w419 {
          frame "False", Default {
          }
          frame "About" {
            n147 = call "Read Exe Version.vi"() -> ("String"=w424:string)  [unwired: 10 in, 1 out]
            n148 = Concatenate Strings("Ice Nucleation Control Software\n\n" ("message"), w424) -> (w425:string)
            n149 = One Button Dialog(message=w425) -> ()  [unwired: 1 in, 1 out]
          }
        }
        n150 = call <vilib>:"Add State(s) to Queue__JKI_lib_State_Machine.vi"("State(s) in (\"\")"=w423) -> ("States Out"=w422:string)  [unwired: 14 in]
      }
      frame "UI: Connections Status" {
        # "Set Status String here\n(this is called takes argument and applies to Status String)"
        n151 = Unbundle By Name(w431) -> ("Connections.cDAQ Therm.Connected"=w430:bool, "Connections.Camera.Connected"=w429:bool, "Connections.cDAQ Voltage.Connected"=w427:bool)
        n152 = call "ConnectionStatus.vi"("cDAQ_AO_status"=w427, "Camera_status"=w429, "cDAQ_Therm_status"=w430) -> ("String"=w428:string)  [unwired: 7 in, 1 out]
        n153 = call <vilib>:"Add State(s) to Queue__JKI_lib_State_Machine.vi"("State(s) in Front (\"\")"=w428, "State(s) in (\"\")"=w434) -> ("States Out"=w433:string)  [unwired: 13 in]
      }
      frame "UI: Start Button" {
        # "Argument"
        # "Set Status String here\n(this is called takes argument and applies to Status String)"
        n154 = case shown="\"Error\"" w438 {
          tunnel: [cluster{u32, u32}[] [{8388608, 8388608}, {4367360, 4367360}, {9342611, 9342611}, {6710891, 6710891}, {16711681, 16711680}, {16711681, 16711680}] ("Colors [4]") cluster{u32, u32}[] [{1985280, 12369084}, {4367360, 4367360}, {8388608, 16711681}, {1985280, 1985280}, {1985280, 4367360}, {8388608, 16711681}] ("Colors [4]") cluster{u32, u32}[] [{1985280, 12369084}, {4367360, 4367360}, {8388608, 16711681}, {1985280, 1985280}, {1985280, 4367360}, {8388608, 16711681}] ("Colors [4]")] -> w437
          tunnel: [string[] ["Error", "Error", "Error", "Error"] ("Strings [4]") string[] ["Ready", "Active", "Stop", "Start"] ("Strings [4]") string[] ["Connecting", "Connecting", "Connecting", "Connecting"] ("Strings [4]")] -> w436
          tunnel: [T8."Enabled" ("Disabled") T8."Enabled" ("Disabled") T8."Disabled" ("Disabled")] -> w435
          frame "Error" {
          }
          frame "Default", Default {
          }
          frame "Connecting" {
          }
        }
        n155 = property on="Start" class="Bool (strict)"("Colors [4]"=w437, "Strings [4]"=w436, "DisabledEnum"=w435) -> ()  [unwired: 2 in, 2 out]
        n156 = call <vilib>:"Add State(s) to Queue__JKI_lib_State_Machine.vi"("State(s) in (\"\")"=w442) -> ("States Out"=w441:string)  [unwired: 14 in]
      }
      frame "UI: Cursor Set" {
        # "Argument"
        # "Set and Unset Cursor Busy.\n(Usage: \"UI: Cursor Set >> Busy|Idle\")"
        n157 = case shown="\"Idle\", Default" w452 {
          tunnel: w454 -> [w459 w461]
          tunnel: [w458 w460] -> w453
          frame "Idle", Default {
            n158 = call <vilib>:"Unset Busy.vi"("error in (no error)"=w459) -> ("error out"=w458:errorcluster)  [unwired: 10 in]
          }
          frame "Busy" {
            n159 = call <vilib>:"Set Busy.vi"("error in (no error)"=w461) -> ("error out"=w460:errorcluster)  [unwired: 9 in, 1 out]
          }
        }
        n160 = call <vilib>:"Add State(s) to Queue__JKI_lib_State_Machine.vi"("State(s) in (\"\")"=w457) -> ("States Out"=w456:string)  [unwired: 14 in]
      }
      frame "UI: Front Panel State" {
        # "Argument"
        # "Set Front Panel Open or Closed\n(Usage: \"UI: Front Panel State >> Open|Close\")"
        n161 = Unbundle By Name(w464) -> ("Core.Current VI Reference"=w463:refnum<vi>)
        n162 = case shown="\"Minimize\", \"Minimized\"" w462 {
          tunnel: w466 -> [w474 w489 w500 w513 w526]
          tunnel: [w476 w490 w502 w515 w528] -> w465
          tunnel: w463 -> [w475 w487 w501 w514 w527]
          frame "Open", "Standard", Default {
            w469 = T5."Standard" ("State")
            n163 = property class="VI"(reference=w475, error in=w474) -> (reference out=w472:refnum<vi>, error out=w473:errorcluster, "FP.State"=w471:T5)
            n164 = Not Equal?(x=w471, y=w469) -> (x != y?=w470:bool)
            n165 = case shown="True" w470 {
              tunnel: [w480 w482] -> w476
              tunnel: w473 -> [w479 w482]
              tunnel: w472 -> [w478 _]
              tunnel: w469 -> [w477 _]
              frame True {
                n166 = invoke class="VI" method="FP.Open"(reference=w478, error in=w479, "Activate"=TRUE, "State"=w477) -> (error out=w480:errorcluster)  [unwired: 1 in, 4 out]
              }
              frame False {
              }
            }
          }
          frame "Close", "Closed" {
            n167 = property class="VI"(reference=w487, error in=w489) -> (reference out=w486:refnum<vi>, error out=w488:errorcluster, "FP.State"=w484:T5)
            n168 = Not Equal?(x=w484, y=T5."Closed" ("Front Panel Window:State")) -> (x != y?=w483:bool)
            n169 = case shown="True" w483 {
              tunnel: [w491 w494] -> w490
              tunnel: w488 -> [w491 w493]
              tunnel: w486 -> [_ w492]
              frame False {
              }
              frame True {
                n170 = invoke class="VI" method="FP.Close"(reference=w492, error in=w493) -> (error out=w494:errorcluster)  [unwired: 1 in, 2 out]
              }
            }
          }
          frame "Hidden", "Hide" {
            w495 = T5."Hidden" ("State")
            n171 = property class="VI"(reference=w501, error in=w500) -> (reference out=w498:refnum<vi>, error out=w499:errorcluster, "FP.State"=w497:T5)
            n172 = Not Equal?(x=w497, y=w495) -> (x != y?=w496:bool)
            n173 = case shown="True" w496 {
              tunnel: [w506 w507] -> w502
              tunnel: w499 -> [w505 w507]
              tunnel: w498 -> [w504 _]
              tunnel: w495 -> [w503 _]
              frame True {
                n174 = invoke class="VI" method="FP.Open"(reference=w504, error in=w505, "State"=w503) -> (error out=w506:errorcluster)  [unwired: 2 in, 4 out]
              }
              frame False {
              }
            }
          }
          frame "Minimize", "Minimized" {
            w508 = T5."Minimized" ("State")
            n175 = property class="VI"(reference=w514, error in=w513) -> (reference out=w511:refnum<vi>, error out=w512:errorcluster, "FP.State"=w510:T5)
            n176 = Not Equal?(x=w510, y=w508) -> (x != y?=w509:bool)
            n177 = case shown="True" w509 {
              tunnel: [w519 w520] -> w515
              tunnel: w512 -> [w518 w520]
              tunnel: w511 -> [w517 _]
              tunnel: w508 -> [w516 _]
              frame True {
                n178 = invoke class="VI" method="FP.Open"(reference=w517, error in=w518, "State"=w516) -> (error out=w519:errorcluster)  [unwired: 2 in, 4 out]
              }
              frame False {
              }
            }
          }
          frame "Maximize", "Maximized" {
            w521 = T5."Maximized" ("State")
            n179 = property class="VI"(reference=w527, error in=w526) -> (reference out=w524:refnum<vi>, error out=w525:errorcluster, "FP.State"=w523:T5)
            n180 = Not Equal?(x=w523, y=w521) -> (x != y?=w522:bool)
            n181 = case shown="True" w522 {
              tunnel: [w532 w533] -> w528
              tunnel: w525 -> [w531 w533]
              tunnel: w524 -> [w530 _]
              tunnel: w521 -> [w529 _]
              frame True {
                n182 = invoke class="VI" method="FP.Open"(reference=w530, error in=w531, "State"=w529) -> (error out=w532:errorcluster)  [unwired: 2 in, 4 out]
              }
              frame False {
              }
            }
          }
        }
        n183 = call <vilib>:"Add State(s) to Queue__JKI_lib_State_Machine.vi"("State(s) in (\"\")"=w468) -> ("States Out"=w467:string)  [unwired: 14 in]
      }
      frame "---------- Macro ----------" {
        # "Do not put any code in this frame.\n(It is a separator no-op. You can make a copy of this frame to create a new Macro frame)"
        n184 = call <vilib>:"Add State(s) to Queue__JKI_lib_State_Machine.vi"("State(s) in (\"\")"=w537) -> ("States Out"=w536:string)  [unwired: 14 in]
      }
      frame "Macro: Initialize" {
        w538 = "UI: StatusString >> Initializing...\nUI: Cursor Set >> Busy\nUI: Start Button >> Connecting\nUI: StatusString >> Initializing Data\nData: Initialize\nUI: StatusString >> Initializing Core Data\nInitialize Core Data\nUI: StatusString >> Loading Calibration File\nData: Load Calibration\nUI: StatusString >> Initializing User Interface\nUI: Initialize\nUI: StatusString >> Initializing Connections\nConnections: Initialize\nUI: Front Panel State >> Open\nUI: Cursor Set >> Idle"  # UI: StatusString >> Initializing... UI: Cursor Set >> Busy UI: Start Button >> Connecting UI: StatusString >> Initializing Data Data: Initialize UI: StatusString >> Initializing Core Data Initialize Core Data UI: StatusString >> Loading Calibration File Data: Load Calibration UI: StatusString >> Initializing User Interface UI: Initialize UI: StatusString >> Initializing Connections Connections: Initialize UI: Front Panel State >> Open UI: Cursor Set >> Idle
        # "Initialization Macro\n(This is called once, when the VI starts)"
        n185 = call <vilib>:"Add State(s) to Queue__JKI_lib_State_Machine.vi"("State(s) in Front (\"\")"=w538, "State(s) in (\"\")"=w542) -> ("States Out"=w541:string)  [unwired: 13 in]
      }
      frame "Macro: Exit" {
        # "Exit Macro\n(This is called once, when the VI exits)"
        n186 = Unbundle By Name(w550) -> ("Core.Close Panel on Exit?"=w549:bool)
        n187 = Select(t="UI: Front Panel State >> Close", s=w549, f="") -> (s? t:f=w546:string)
        n188 = call <vilib>:"Add State(s) to Queue__JKI_lib_State_Machine.vi"("State(s) in Front (\"\")"="UI: StatusString >> Closing System... Terminating Data Acquisition\nSystem: Stop\nUI: StatusString >> Closing System... Terminating Connections\nConnections: Terminate\nUI: StatusString >> Closing System... Data Cleanup\nData: Cleanup\nUI: StatusString >> Closing System" ("State(s) in Front (\"\")"), "State(s) in (\"\")"=w546, "State(s) at Back (\"\")"="Exit") -> ("States Out"=w545:string)  [unwired: 12 in]
        n189 = call <vilib>:"Add State(s) to Queue__JKI_lib_State_Machine.vi"("State(s) in Front (\"\")"=w545, "State(s) in (\"\")"=w553) -> ("States Out"=w552:string)  [unwired: 13 in]
      }
      frame "---------- System ----------" {
        # "Template Separator\n(You can make a copy of, or modify, this frame)"
        n190 = call <vilib>:"Add State(s) to Queue__JKI_lib_State_Machine.vi"("State(s) in (\"\")"=w557) -> ("States Out"=w556:string)  [unwired: 14 in]
      }
      frame "System: Start" {
        # "Your code here.\n(You can make a copy of, or modify, this frame)"
        n191 = Unbundle By Name(w558) -> ("Data Acquisition.Ready"=w560:bool, "Data Acquisition.Active"=w561:bool)
        n192 = Not(x=w561) -> (.not. x?=w559:bool)
        n193 = And(x=w560, y=w559) -> (x .and. y?=w562:bool)
        n194 = case shown="True" w562 {
          selector: w562 -> [w569 _]
          tunnel: [w568 "UI: Cursor Set >> Busy \nUI: StatusString >> Clearing Chart\nUI: Chart Setup\nUI: Chart Clear\n// ----------- Data Files Setup ----------- //\nUI: StatusString >> Configuring Setup file\nData: Setup File Config\nUI: StatusString >> Configuring Data file\nData: Data File Config\nUI: StatusString >> Configuring Image Folder\nData: Image Folder Setup\n// ----------- Data Acquisition Setup----------- //\nUI: StatusString >> Initializing Buffer\nData Acquisition: Buffer Initialize\nUI: StatusString >> Initializing cDAQ\nData Acquisition: cDAQ Initialize\nData Acquisition: cDAQ AO Initialize\nUI: StatusString >> Initializing Camera\nData Acquisition: Camera Initialize\nData Acquisition: Start\nUI: StatusString >> System Active\nUI: Cursor Set >> Idle" ("State(s) in Front (\"\")")] -> w563
          tunnel: w560 -> [w567 _]
          frame False {
            n195 = local write "Start"(w569) -> ()
            n196 = case shown="False" w567 {
              tunnel: ["UI: Connections Status" ("State(s) in Front (\"\")") "" ("State(s) in Front (\"\")")] -> w568
              frame False {
              }
              frame True {
              }
            }
          }
          frame True {
          }
        }
        n197 = call <vilib>:"Add State(s) to Queue__JKI_lib_State_Machine.vi"("State(s) in Front (\"\")"=w563, "State(s) in (\"\")"=w566) -> ("States Out"=w565:string)  [unwired: 13 in]
      }
      frame "System: Override" {
        # "Your code here.\n(You can make a copy of, or modify, this frame)"
        n198 = Bundle By Name(cluster=w576, "Data Acquisition.Ready"=TRUE ("System.Active")) -> (w575:T2)
        n199 = call <vilib>:"Add State(s) to Queue__JKI_lib_State_Machine.vi"("State(s) in Front (\"\")"="UI: Start Button >> Default" ("State(s) in Front (\"\")"), "State(s) in (\"\")"=w579) -> ("States Out"=w578:string)  [unwired: 13 in]
      }
      frame "System: Stop" {
        # "Your code here.\n(You can make a copy of, or modify, this frame)"
        n200 = Unbundle By Name(w581) -> ("Data Acquisition.Active"=w582:bool)
        n201 = case shown="True" w582 {
          tunnel: ["" ("State(s) in Front (\"\")") "UI: Cursor Set >> Busy\nUI: StatusString >> Terminating cDAQ\nData Acquisition: cDAQ Terminate\nData Acquisition: cDAQ AO Terminate\nUI: StatusString >> Terminating Camera\nData Acquisition: Camera Terminate\nUI: StatusString >> Terminating Buffer\nData Acquisition: Buffer Terminate\nUI: StatusString >> Unlocking files\nData: Files Unlock\nUI: StatusString >> Stamping Times\nData: Stamp times\nUI: StatusString >> Idle\nUI: Cursor Set >> Idle" ("State(s) in Front (\"\")")] -> w583
          tunnel: w581 -> [w588 w590]
          tunnel: [w588 w589] -> w580
          frame False {
          }
          frame True {
            n202 = Bundle By Name(cluster=w590, "Data Acquisition.Active"=FALSE ("System.Active")) -> (w589:T2)
          }
        }
        n203 = call <vilib>:"Add State(s) to Queue__JKI_lib_State_Machine.vi"("State(s) in Front (\"\")"=w583, "State(s) in (\"\")"=w586) -> ("States Out"=w585:string)  [unwired: 13 in]
      }
      frame "---------- Data Acquisition ----------" {
        # "Template Separator\n(You can make a copy of, or modify, this frame)"
        n204 = call <vilib>:"Add State(s) to Queue__JKI_lib_State_Machine.vi"("State(s) in (\"\")"=w596) -> ("States Out"=w595:string)  [unwired: 14 in]
      }
      frame "Data Acquisition: cDAQ Initialize" {
        # "Your code here.\n(You can make a copy of, or modify, this frame)"
        n205 = Unbundle By Name(w602) -> ("Connections.cDAQ Therm.Task"=w605:refnum<k21>, "Connections.cDAQ Therm.Connected"=w600:bool, "Connections.cDAQ Therm.Active"=w598:bool)
        n206 = Not(x=w598) -> (.not. x?=w597:bool)
        n207 = And(x=w600, y=w597) -> (x .and. y?=w599:bool)
        n208 = case shown="True" w599 {
          tunnel: w605 -> [_ w615]
          tunnel: w604 -> [w608 w614]
          tunnel: [w608 w613] -> w603
          tunnel: w602 -> [w609 w611]
          tunnel: [w609 w610] -> w601
          frame False {
          }
          frame True {
            n209 = Bundle By Name(cluster=w611, "Connections.cDAQ Therm.Active"=TRUE ("Connections.Camera.Active")) -> (w610:T2)
            n210 = call <vilib>:"DAQmx Start Task.vi"("task/channels in"=w615, "error in"=w614) -> ("error out"=w613:errorcluster)  [unwired: 12 in, 1 out]
          }
        }
        n211 = call <vilib>:"Add State(s) to Queue__JKI_lib_State_Machine.vi"("State(s) in (\"\")"=w607) -> ("States Out"=w606:string)  [unwired: 14 in]
      }
      frame "Data Acquisition: cDAQ Terminate" {
        # "Your code here.\n(You can make a copy of, or modify, this frame)"
        n212 = Unbundle By Name(w618) -> ("Connections.cDAQ Therm.Task"=w621:refnum<k21>, "Connections.cDAQ Therm.Connected"=w616:bool)
        n213 = case shown="True" w616 {
          tunnel: w621 -> [_ w631]
          tunnel: w620 -> [w624 w630]
          tunnel: [w624 w629] -> w619
          tunnel: w618 -> [w625 w627]
          tunnel: [w625 w626] -> w617
          frame False {
          }
          frame True {
            n214 = Bundle By Name(cluster=w627, "Connections.cDAQ Therm.Active"=FALSE ("Connections.Camera.Active")) -> (w626:T2)
            n215 = call <vilib>:"DAQmx Stop Task.vi"("task/channels in"=w631, "error in"=w630) -> ("error out"=w629:errorcluster)  [unwired: 12 in, 1 out]
          }
        }
        n216 = call <vilib>:"Add State(s) to Queue__JKI_lib_State_Machine.vi"("State(s) in (\"\")"=w623) -> ("States Out"=w622:string)  [unwired: 14 in]
      }
      frame "Data Acquisition: cDAQ AO Initialize" {
        # "Your code here.\n(You can make a copy of, or modify, this frame)"
        n217 = Unbundle By Name(w634) -> ("Connections.cDAQ Voltage.Task"=w637:refnum<k21>, "Connections.cDAQ Voltage.Connected"=w632:bool)
        n218 = case shown="True" w632 {
          tunnel: w637 -> [_ w647]
          tunnel: w636 -> [w640 w646]
          tunnel: [w640 w645] -> w635
          tunnel: w634 -> [w641 w643]
          tunnel: [w641 w642] -> w633
          frame False {
          }
          frame True {
            n219 = Bundle By Name(cluster=w643, "Connections.cDAQ Voltage.Active"=TRUE ("Connections.Camera.Active")) -> (w642:T2)
            n220 = call <vilib>:"DAQmx Start Task.vi"("task/channels in"=w647, "error in"=w646) -> ("error out"=w645:errorcluster)  [unwired: 12 in, 1 out]
          }
        }
        n221 = call <vilib>:"Add State(s) to Queue__JKI_lib_State_Machine.vi"("State(s) in (\"\")"=w639) -> ("States Out"=w638:string)  [unwired: 14 in]
      }
      frame "Data Acquisition: cDAQ AO Terminate" {
        # "Your code here.\n(You can make a copy of, or modify, this frame)"
        n222 = Unbundle By Name(w650) -> ("Connections.cDAQ Voltage.Task"=w653:refnum<k21>, "Connections.cDAQ Voltage.Connected"=w648:bool)
        n223 = case shown="True" w648 {
          tunnel: w653 -> [_ w662]
          tunnel: w652 -> [w656 w659]
          tunnel: [w656 w666] -> w651
          tunnel: w650 -> [w657 w664]
          tunnel: [w657 w663] -> w649
          frame False {
          }
          frame True {
            n224 = Bundle By Name(cluster=w664, "Connections.cDAQ Voltage.Active"=FALSE ("Connections.Camera.Active")) -> (w663:T2)
            n225 = call-poly <vilib>:"DAQmx Write.vi"("task/channels in"=w662, "data"=0.0, "error in"=w659) -> ("task out"=w661:refnum<k21>, "error out"=w660:errorcluster)  [unwired: 10 in, 1 out]
            n226 = call <vilib>:"DAQmx Stop Task.vi"("task/channels in"=w661, "error in"=w660) -> ("error out"=w666:errorcluster)  [unwired: 12 in, 1 out]
          }
        }
        n227 = call <vilib>:"Add State(s) to Queue__JKI_lib_State_Machine.vi"("State(s) in (\"\")"=w655) -> ("States Out"=w654:string)  [unwired: 14 in]
      }
      frame "Data Acquisition: Camera Initialize" {
        # "Your code here.\n(You can make a copy of, or modify, this frame)"
        n228 = Unbundle By Name(w668) -> ("Connections.Camera.Connected"=w667:bool)
        n229 = case shown="True" w667 {
          tunnel: [w674 w680] -> w671
          tunnel: w670 -> [w675 w679]
          tunnel: [w675 w678] -> w669
          tunnel: w668 -> [w674 w677]
          frame False {
          }
          frame True {
            n230 = call "Camera_Config.vi"("error in (no error)"=w679, "crop?"=TRUE, "DataCluster in"=w677) -> ("error out"=w678:errorcluster, "DataCluster out"=w680:T2)  [unwired: 7 in]
          }
        }
        n231 = call <vilib>:"Add State(s) to Queue__JKI_lib_State_Machine.vi"("State(s) in (\"\")"=w673) -> ("States Out"=w672:string)  [unwired: 14 in]
      }
      frame "Data Acquisition: Camera Terminate" {
        # "Your code here.\n(You can make a copy of, or modify, this frame)"
        n232 = Unbundle By Name(w685) -> ("Data Acquisition.Camera.Image"=w682:T1, "Connections.Camera.Session"=w687:T3, "Connections.Camera.Connected"=w683:bool)
        n233 = case shown="True" w683 {
          tunnel: w687 -> [_ w701]
          tunnel: w686 -> [w690 w700]
          tunnel: w685 -> [w691 w699]
          tunnel: [w691 w697] -> w684
          tunnel: w682 -> [_ w694]
          tunnel: [w690 w692] -> w681
          frame False {
          }
          frame True {
            n234 = call <vilib>:"IMAQdx Unconfigure Acquisition.vi"("error in"=w700, "Session In"=w701) -> ("error out"=w696:errorcluster, "Session Out"=w695:T3)  [unwired: 8 in]
            n235 = Bundle By Name(cluster=w699, "Connections.Camera.Active"=FALSE) -> (w697:T2)
            n236 = call <vilib>:"IMAQdx Stop Acquisition.vi"("error in"=w696, "Session In"=w695) -> ("error out"=w693:errorcluster)  [unwired: 8 in, 1 out]
            n237 = call "IMAQ Dispose"("Image"=w694, "error in (no error)"=w693) -> ("error out"=w692:errorcluster)  [unwired: 4 in]
          }
        }
        n238 = call <vilib>:"Add State(s) to Queue__JKI_lib_State_Machine.vi"("State(s) in (\"\")"=w689) -> ("States Out"=w688:string)  [unwired: 14 in]
      }
      frame "Data Acquisition: Buffer Initialize" {
        # "Access Data Setup here.\n(this is called automatically, by the Settings Event Run time menu)"
        n239 = call "Buffer_Initialize.vi"("error in (no error)"=w704, "DataCluster in"=w705) -> ("error out"=w703:errorcluster, "DataCluster Out"=w702:T2)  [unwired: 8 in]
        n240 = call <vilib>:"Add State(s) to Queue__JKI_lib_State_Machine.vi"("State(s) in (\"\")"=w707) -> ("States Out"=w706:string)  [unwired: 14 in]
      }
      frame "Data Acquisition: Buffer Terminate" {
        # "Access Data Setup here.\n(this is called automatically, by the Settings Event Run time menu)"
        n241 = Unbundle By Name(w708) -> ("Data Acquisition.Queue.Queue"=w709:refnum<queue>)
        n242 = Release Queue(queue=w709, force destroy? (F)=FALSE, error in (no error)=w711) -> (error out=w710:errorcluster)  [unwired: 2 out]
        n243 = call <vilib>:"Add State(s) to Queue__JKI_lib_State_Machine.vi"("State(s) in (\"\")"=w714) -> ("States Out"=w713:string)  [unwired: 14 in]
      }
      frame "Data Acquisition: Start" {
        # "Access Data Setup here.\n(this is called automatically, by the Settings Event Run time menu)"
        n244 = Unbundle By Name(w715) -> ("Data Acquisition.Ready"=w721:bool, "Data Acquisition.Active"=w720:bool)
        n245 = Not(x=w720) -> (.not. x?=w722:bool)
        n246 = And(x=w721, y=w722) -> (x .and. y?=w716:bool)
        n247 = case shown="True" w716 {
          selector: w716 -> [w728 _]
          tunnel: [w727 _] -> w718
          tunnel: w715 -> [w726 w733]
          tunnel: [w726 w731] -> w719
          tunnel: w721 -> [w725 _]
          frame False {
            n248 = local write "Start"(w728) -> ()
            n249 = case shown="True" w725 {
              tunnel: ["UI: Connections Status" ("State(s) in Front (\"\")") "" ("State(s) in Front (\"\")")] -> w727
              frame False {
              }
              frame True {
              }
            }
          }
          frame True {
            n250 = Bundle By Name(cluster=w733, "Data Acquisition.Active"=TRUE ("System.Active")) -> (w731:T2)
          }
        }
        n251 = call <vilib>:"Add State(s) to Queue__JKI_lib_State_Machine.vi"("State(s) in Front (\"\")"=w718, "State(s) in (\"\")"=w724) -> ("States Out"=w723:string)  [unwired: 13 in]
      }
      frame "---------- Tools ----------" {
        # "Template Separator\n(You can make a copy of, or modify, this frame)"
        n252 = call <vilib>:"Add State(s) to Queue__JKI_lib_State_Machine.vi"("State(s) in (\"\")"=w737) -> ("States Out"=w736:string)  [unwired: 14 in]
      }
      frame "Tools: Sensor Readout" {
        # "Your code here.\n(You can make a copy of, or modify, this frame)"
        n253 = call "Thermistor_Manual_Read.vi"("error in"=w741, "temp readings"=w739, "input cluster"=w742) -> ("error out"=w740:errorcluster, "state"=w738:string)  [unwired: 7 in]
        n254 = call <vilib>:"Add State(s) to Queue__JKI_lib_State_Machine.vi"("State(s) in Front (\"\")"=w738, "State(s) in (\"\")"=w744) -> ("States Out"=w743:string)  [unwired: 13 in]
      }
      frame "Tools: Camera Feed" {
        # "Your code here.\n(You can make a copy of, or modify, this frame)"
        n255 = call "Camera_Feed.vi"("error in"=w747, "DataCluster"=w748) -> ("error out"=w746:errorcluster, "State out"=w745:string)  [unwired: 7 in, 1 out]
        n256 = call <vilib>:"Add State(s) to Queue__JKI_lib_State_Machine.vi"("State(s) in Front (\"\")"=w745, "State(s) in (\"\")"=w750) -> ("States Out"=w749:string)  [unwired: 13 in]
      }
      frame "Tools: Manual Temp Control" {
        # "Your code here.\n(You can make a copy of, or modify, this frame)"
        n257 = call "Manual_Cool_Heat.vi"("error in"=w754, "input cluster"=w755) -> ("error out"=w753:errorcluster, "State out"=w752:string, "input cluster out"=w751:T2)  [unwired: 7 in]
        n258 = call <vilib>:"Add State(s) to Queue__JKI_lib_State_Machine.vi"("State(s) in Front (\"\")"=w752, "State(s) in (\"\")"=w757) -> ("States Out"=w756:string)  [unwired: 13 in]
      }
      frame "Tools: Freeze Check" {
        # "Access Data Setup here.\n(this is called automatically, by the Settings Event Run time menu)"
        n259 = call "Freeze_Check.vi"("DataCluster in"=w758) -> ()  [unwired: 10 in, 1 out]
        n260 = call <vilib>:"Add State(s) to Queue__JKI_lib_State_Machine.vi"("State(s) in (\"\")"=w761) -> ("States Out"=w760:string)  [unwired: 14 in]
      }
    }
    n261 = call <extravilib>:"Read.vi"("channel"=w9) -> ("element"=w8:string)  [unwired: 1 in, 1 out]
    n262 = call <vilib>:"Add State(s) to Queue__JKI_lib_State_Machine.vi"("State(s) in Front (\"\")"=w8, "State(s) in (\"\")"=w11) -> ("States Out"=w10:string)  [unwired: 13 in]
    n263 = call <extravilib>:"Write.vi"("element"=w13) -> ("channel"=w12:T10)  [unwired: 1 out]
  }
  n264 = while "Data Acquisition Loop" {
    tunnel: w3 -> [w768]
    tunnel: w3 -> [w767]
    tunnel: [w763] -> w2
    tunnel: [w762] -> w1
    stop <- w766 stop-if-true
    n265 = call <extravilib>:"Read.vi"("channel"=w768) -> ("element"=w764:T2)  [unwired: 1 in, 1 out]
    n266 = call "SystemActive.vi"("DataCluster"=w764) -> ("Active"=w765:bool, "Exit"=w766:bool)  [unwired: 1 in, 2 out]
    n267 = case shown="True" w765 {
      tunnel: w767 -> [_ w779]
      tunnel: w764 -> [_ w776]
      tunnel: [_ w771] -> w763
      tunnel: [_ w770] -> w762
      frame False {
        # "Data Acquisition Idle"
        n268 = Wait (ms)(milliseconds to wait=u32 100) -> ()  [unwired: 1 out]
      }
      frame True {
        # "Data Acquisition Active"
        n269 = call "SampleRate_Convert.vi"("DataCluster"=w776) -> ("Sample dt (ms)"=w775:i64)  [unwired: 5 in, 3 out]
        n270 = node-c288(w775) -> (w778:T11)
        n271 = timed-loop {
          tunnel: w779 -> [w805]
          timing: w778 -> [_]
          timing-out: [_] -> w777
          shift-right: [w802] -> _
          shift-left: cluster{dbl[], dbl[], dbl[], dbl[], dbl[][]} {[], [], [], [], []} ("Data Cluster in") -> [w801]
          shift-right: [w787] -> _
          shift-left: 0.0 ("Mean Temperature") -> [w800]
          shift-right: [FALSE] -> _
          shift-left: TRUE -> [w793]
          tunnel: [w785] -> w771
          tunnel: [w781] -> w770
          stop <- w804 stop-if-true
          w798 = u16 0 items=["DAQ", "Control"] ("DAQ/Control")
          n272 = node-c288() -> (→"Period (ms)":i64)  [unwired: 1 in]
          n273 = call <extravilib>:"Read.vi"("channel"=w805) -> ("element"=w794:T2)  [unwired: 1 in, 1 out]
          n274 = call "cDAQ_Read.vi"("Prev Temp"=w800, "DAQ/Control"=w798, "DataCluster"=w794) -> ("Temp Gradient"=w791:dbl, "Mean Temperature"=w787:dbl, "Temperature Readings"=w796:dbl[], "Voltage Readings"=w803:dbl[], "valid sample?"=w799:bool)  [unwired: 3 in, 1 out]
          n275 = call "SystemActive.vi"("current temp"=w787, "DataCluster"=w794) -> ("!Active/Exit"=w804:bool, "Temp reached"=w786:bool)  [unwired: 2 out]
          n276 = call "Camera_Grab.vi"("DataCluster"=w794) -> ("Image Out"=w795:T1)  [unwired: 9 in, 1 out]
          "Camera Feed" <- w795
          n277 = call "PID_Control.vi"("DataCluster"=w794, "Gradient"=w791, "PID"=TRUE, "reinitialize? (F)"=w793) -> ("Output%"=→"Output%":dbl)  [unwired: 8 in, 3 out]
          n278 = call "Chart_Data_Packer.vi"("DataCluster"=w794, "Mean Temperature"=w787, "Temperatures"=w796, "Temp Gradient"=w791, "Data Cluster in"=w801, "DAQ/Control"=w798) -> ("Gradients"=→"Gradients":waveform(dbl)[], "Temps"=→"Temps":waveform(dbl)[], "Data Cluster"=w802:cluster{dbl[], dbl[], dbl[], dbl[], dbl[][]})  [unwired: 6 in, 1 out]
          n279 = call "Buffer_Append.vi"("DataCluster"=w794, "Log?"=w799, "Image Out"=w795, "Voltage Readings"=w803, "Temperature Readings"=w796) -> ("Temperature Readings Duplicate"=w784:dbl[], "Voltage Readings Duplicate"=w783:dbl[])  [unwired: 9 in]
          n280 = case shown="True" w786 {
            tunnel: [_ w806] -> w785
            frame False {
            }
            frame True {
              n281 = call <extravilib>:"Write.vi"("element"="System: Stop") -> ("channel"=w806:T14)  [unwired: 1 out]
            }
          }
          n282 = node-c288() -> ()  [unwired: 1 out]
          n283 = Bundle("Temperature Readings Duplicate"=w784, "Voltage Readings Duplicate"=w783) -> (w782:T15)  [unwired: 1 in]
          n284 = call <extravilib>:"Write.vi"("element"=w782) -> ("channel"=w781:T16)  [unwired: 1 out]
        }
        n285 = node-c288(w777) -> ()
      }
    }
  }
  n286 = while "Data Logging Loop" {
    tunnel: w3 -> [w820]
    tunnel: w3 -> [w819]
    stop <- w818 stop-if-true
    n287 = call <extravilib>:"Read.vi"("channel"=w820) -> ("element"=w816:T2)  [unwired: 1 in, 1 out]
    n288 = call "SystemActive.vi"("DataCluster"=w816) -> ("Active"=w817:bool, "Exit"=w818:bool)  [unwired: 1 in, 2 out]
    n289 = call "Camera_Frequency.vi"("DataCluster"=w816) -> ("Image Frequency"=w815:i32)
    n290 = case shown="True" w817 {
      tunnel: w819 -> [_ w823]
      tunnel: w815 -> [_ w822]
      frame False {
        # "Data Acquisition Idle"
        n291 = Wait (ms)(milliseconds to wait=u32 100) -> ()  [unwired: 1 out]
      }
      frame True {
        # "Data Acquisition Active"
        n292 = while {
          tunnel: w823 -> [w829]
          shift-right: [w824] -> _
          shift-left: w822 -> [w825]
          stop <- w828 stop-if-true
          # "Active Data Logging Loop"
          n293 = call <extravilib>:"Read.vi"("channel"=w829) -> ("element"=w826:T2)  [unwired: 1 in, 1 out]
          n294 = call "SystemActive.vi"("DataCluster"=w826) -> ("!Active/Exit"=w828:bool)  [unwired: 1 in, 3 out]
          n295 = call "DataFile_Append.vi"("iteration"=w825, "DataCluster"=w826) -> ("iteration out"=w824:i32)  [unwired: 9 in]
          n296 = Wait (ms)(milliseconds to wait=u32 50) -> ()  [unwired: 1 out]
        }
      }
    }
  }
